vi "单参数加标流程.vi"(10 "流程类型":T3, 11 "Slave ID":T5=enum."氨氮") -> ()   [LabVIEW 2016, in "质控单元V2.lvlib"]
panel:
  in  "平行样测试数据":T1={"时间"=timestamp(0 s since 1904-01-01), "参数"="", "数据类型"="N", "第一次水样浓度值"=0.0, "第二次水样测试时间"=timestamp(0 s since 1904-01-01), "第二次水样浓度值"=0.0}
  in  "集成干预测试数据":T2={"时间"=timestamp(0 s since 1904-01-01), "参数"="", "数据类型"="N", "集成干预测试浓度值"=0.0, "集成干预前测试时间"=timestamp(0 s since 1904-01-01), "集成干预前测试浓度值"=0.0}
  out "平行样启动时间":timestamp
  in  "获取加标回收测试数据计数":u16
  in  "获取水样测试数据计数":u16
  in  "写入加标体积重试次数":u16
  in  "加标模块加标润洗启动计数":u16
  out "加标回收启动时间":timestamp
  out "水样测试启动时间":timestamp
  out "Next State":string
  in  "仪器加标回收启动计数":u16
  in  "仪器水样测试启动计数":u16
  in  "加标模块排液启动计数":u16
  in  "加标模块加标启动计数":u16
  in  "加标模块进样启动计数":u16
  in  "加标模块水样润洗启动计数":u16
  in  "采配水启动次数计数":u16
  in  "加标回收测试时间":timestamp
  in  "水样测试时间":timestamp
  in  "质控数据":T4
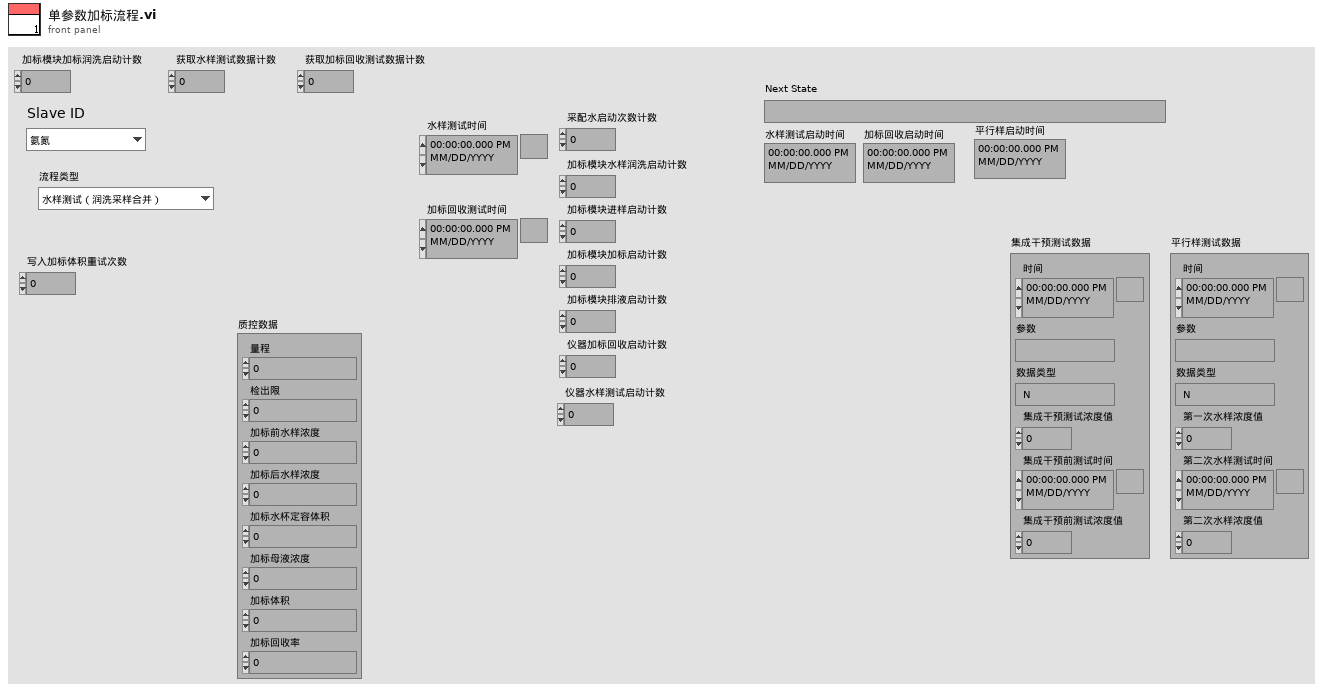
[diagram p1: front panel]
types:
  T1 = typedef "平行样测试数据字段定义.ctl" = cluster{"时间":timestamp, "参数":string, "数据类型":string, "第一次水样浓度值":dbl, "第二次水样测试时间":timestamp, "第二次水样浓度值":dbl}
  T2 = typedef "集成干预字段定义.ctl" = cluster{"时间":timestamp, "参数":string, "数据类型":string, "集成干预测试浓度值":dbl, "集成干预前测试时间":timestamp, "集成干预前测试浓度值":dbl}
  T3 = typedef "质控单元V2.lvlib/测试子流程.ctl" = enum16{"水样测试（润洗采样合并）", "水样测试（不启动采配水）", "加标回收（润洗采样合并）", "加标回收（不启动采配水）", "集成干预测试", "平行样测试", "平行样测试（不启动采配水）", "水样测试（不含采样杯）", "平行样测试（不含采样杯）", "集成干预测试（不含采样杯）"}
  T4 = cluster{"量程":dbl, "检出限":dbl, "加标前水样浓度":dbl, "加标后水样浓度":dbl, "加标水杯定容体积":dbl, "加标母液浓度":dbl, "加标体积":dbl, "加标回收率":dbl}
  T5 = typedef "质控单元V2.lvlib/质控slave id.ctl" = enum16{"null", "氨氮", "总磷", "总氮", "CODMn", "CODCr"}
  T6 = cluster{"氨氮":bool, "总磷":bool, "总氮":bool, "CODMn":bool, "CODCr":bool}
  T7 = cluster{"时间":timestamp, "参数":string, "数据类型":string, "加标回收率":sgl, "加标前水样测试时间":timestamp, "加标前水样浓度值":sgl, "加标后水样浓度值":sgl, "加标母液浓度值":sgl, "加标体积":sgl, "加标水杯定容体积":sgl}
  T8 = enum16{"待机", "水样测试（全流程）", "停止", "加标回收", "水样测试（简易流程）"}
  T9 = enum16{"待机", "润洗", "采样", "沉淀", "配水", "反冲洗", "储水", "结束"}
  T10 = typedef "质控单元V2.lvlib/采配水通用流程.ctl" = enum16{"待机", "润洗", "采样", "沉淀", "配水", "反冲洗", "结束"}
  T11 = typedef "质控单元V2.lvlib/质控流程控制.ctl" = enum16{"待机", "启动进样流程", "启动加标流程", "启动排液流程", "停止流程", "加标（单独一步骤）"}
  T12 = enum16{"待机", "润洗", "进样", "定量", "加标", "等待取样", "排液", "异常停机"}
  T13 = enum16{"空闲", "水样测试", "标样核查", "零点核查", "跨度核查", "空白测试", "平行样测试", "加标回收", "空白校准", "标样校准", "初始化（清洗）"}
  T14 = cluster{"时间":timestamp, "参数":string, "数据类型":string, "第一次水样浓度值":dbl, "第二次水样测试时间":timestamp, "第二次水样浓度值":dbl}
  T15 = cluster{"水样数据时间":timestamp, "水样实测值":sgl, "水样数据标识":string}
  T16 = cluster{"加标回收数据时间":timestamp, "加标回收实测值":sgl, "加标回收数据标识":string}
  T17 = typedef "质控单元V2.lvlib/质控仪器状态.ctl" = cluster{"运行状态":enum16{"待机", "润洗", "进样", "定量", "加标", "等待取样", "排液"}, "液位状态":enum16{"无感应", "有感应"}, "告警状态":enum16{"无告警", "液位故障告警", "注射泵异常"}, "当前步骤数":u16, "当前步骤剩余时间":u16, "当前步骤具体操作":enum16{"加标", "进样", "排液", "搅拌", "定量"}, "当前流程":enum16{"待机", "进样流程", "加标流程", "排液流程"}}
  T18 = enum16{"待机", "润洗", "进样", "定量", "加标", "等待取样", "排液"}
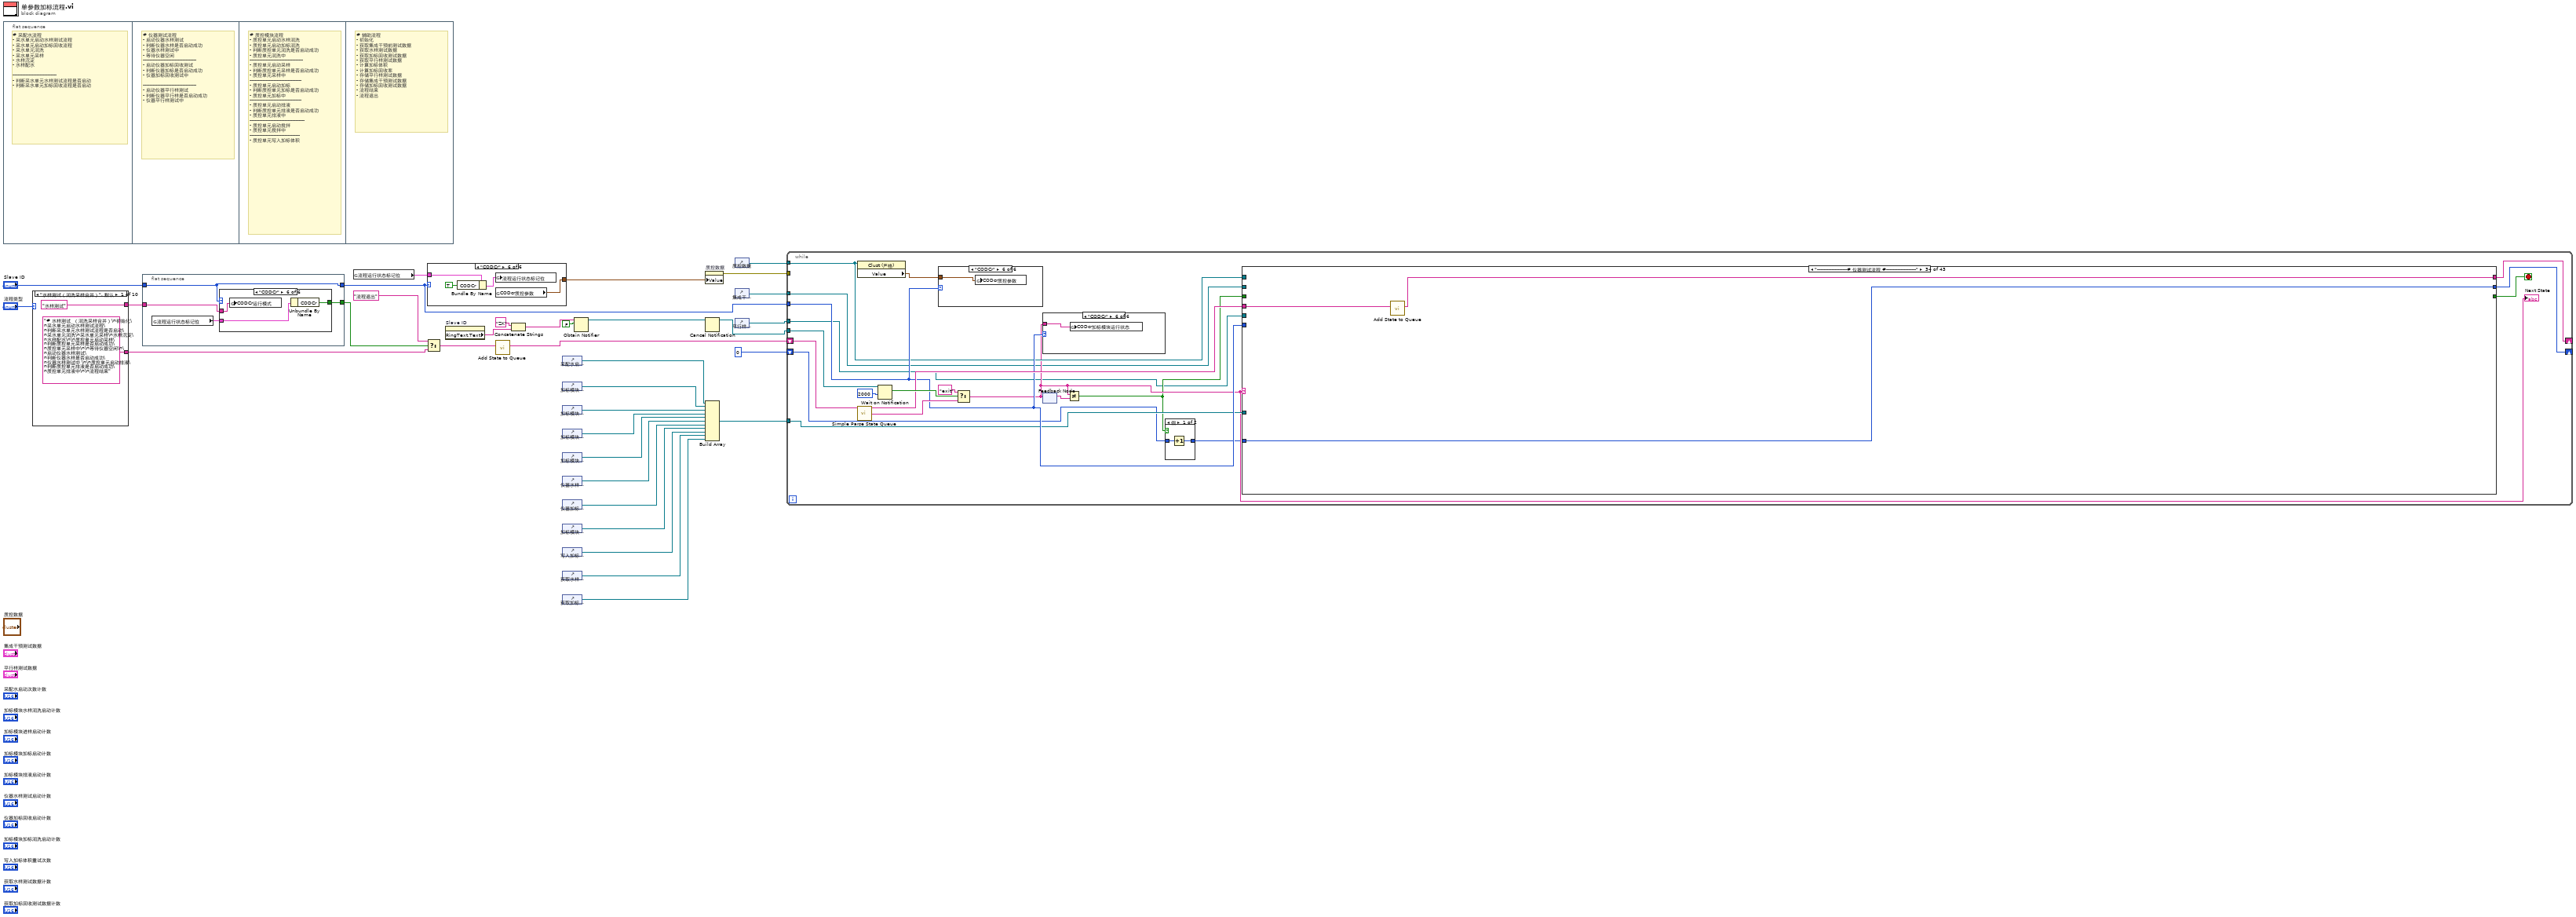
[diagram p0: block diagram]
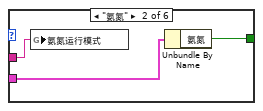
[diagram p3: hidden frame]
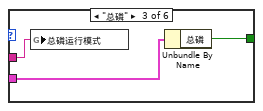
[diagram p4: hidden frame]
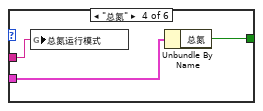
[diagram p5: hidden frame]
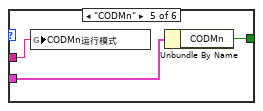
[diagram p6: hidden frame]
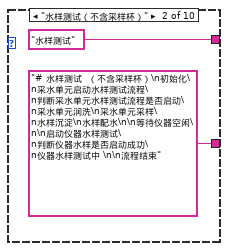
[diagram p7: hidden frame]
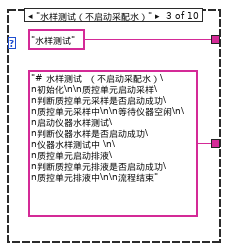
[diagram p8: hidden frame]
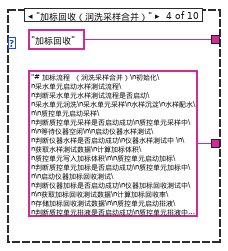
[diagram p9: hidden frame]
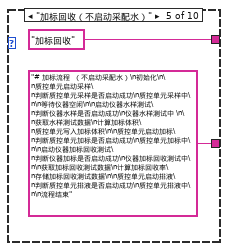
[diagram p10: hidden frame]
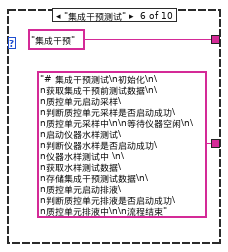
[diagram p11: hidden frame]
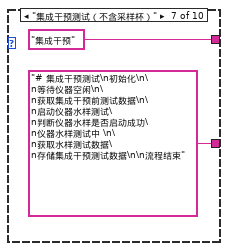
[diagram p12: hidden frame]
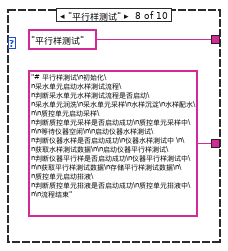
[diagram p13: hidden frame]
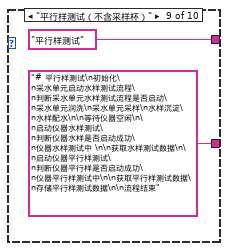
[diagram p14: hidden frame]
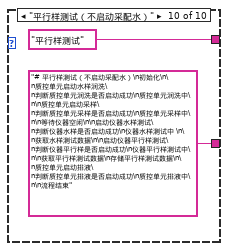
[diagram p15: hidden frame]
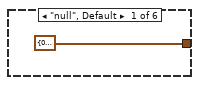
[diagram p16: hidden frame]
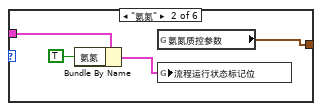
[diagram p17: hidden frame]
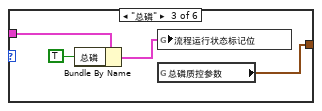
[diagram p18: hidden frame]
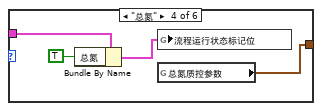
[diagram p19: hidden frame]
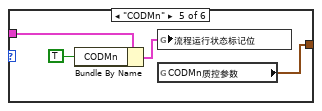
[diagram p20: hidden frame]
diagram:
  n1 = flat-sequence {
    frame #0 {
      # "# 采配水流程\n- 采水单元启动水样测试流程\n- 采水单元启动加标回收流程\n- 采水单元润洗\n- 采水单元采样 \n- 水样沉淀\n- 水样配水\n\n----------------------------\n- 判断采水单元水样测试流程是否启动\n- 判断采水单元加标回收流程是否启动"
    }
    frame #1 {
      # "# 仪器测试流程\n- 启动仪器水样测试\n- 判断仪器水样是否启动成功\n- 仪器水样测试中\n- 等待仪器空闲\n----------------------------------\n- 启动仪器加标回收测试\n- 判断仪器加标是否启动成功\n- 仪器加标回收测试中\n\n----------------------------------\n- 启动仪器平行样测试\n- 判断仪器平行样是否启动成功\n- 仪器平行样测试中"
    }
    frame #2 {
      # "# 质控模块流程\n- 质控单元启动水样润洗\n- 质控单元启动加标润洗\n- 判断质控单元润洗是否启动成功\n- 质控单元润洗中\n----------------------------------\n- 质控单元启动采样\n- 判断质控单元采样是否启动成功\n- 质控单元采样中\n---------------------------------\n- 质控单元启动加标\n- 判断质控单元加标是否启动成功\n- 质控单元加标中\n---------------------------------\n- 质控单元启动排液\n- 判断质控单元排液是否启动成功\n- 质控单元排液中\n-----------------------------------\n- 质控单元启动搅拌\n- 质控单元搅拌中\n--------------------------------\n- 质控单元写入加标体积"
    }
    frame #3 {
      # "# 辅助流程\n- 初始化\n- 获取集成干预前测试数据\n- 获取水样测试数据\n- 获取加标回收测试数据\n- 获取平行样测试数据\n- 计算加标体积\n- 计算加标回收率\n- 存储平行样测试数据\n- 存储集成干预测试数据\n- 存储加标回收测试数据 \n- 流程结束\n- 流程退出"
    }
  }
  n2 = case shown="\"水样测试（润洗采样合并）\", 默认" "流程类型" {
    tunnel: ["# 水样测试  （润洗采样合并）\n初始化\n采水单元启动水样测试流程\n判断采水单元水样测试流程是否启动\n采水单元润洗\n采水单元采样\n水样沉淀\n水样配水\n\n质控单元启动采样\n判断质控单元采样是否启动成功\n质控单元采样中\n\n等待仪器空闲\n\n启动仪器水样测试\n判断仪器水样是否启动成功\n仪器水样测试中 \n\n质控单元启动排液\n判断质控单元排液是否启动成功\n质控单元排液中\n\n流程结束" ("State(s) In (\"\")") "# 水样测试  （不含采样杯）\n初始化\n采水单元启动水样测试流程\n判断采水单元水样测试流程是否启动\n采水单元润洗\n采水单元采样\n水样沉淀\n水样配水\n\n等待仪器空闲\n\n启动仪器水样测试\n判断仪器水样是否启动成功\n仪器水样测试中 \n\n流程结束" ("State(s) In (\"\")") "# 水样测试  （不启动采配水）\n初始化\n\n质控单元启动采样\n判断质控单元采样是否启动成功\n质控单元采样中\n\n等待仪器空闲\n\n启动仪器水样测试\n判断仪器水样是否启动成功\n仪器水样测试中 \n\n质控单元启动排液\n判断质控单元排液是否启动成功\n质控单元排液中\n\n流程结束" ("State(s) In (\"\")") "# 加标流程  （润洗采样合并）\n初始化\n采水单元启动水样测试流程\n判断采水单元水样测试流程是否启动\n采水单元润洗\n采水单元采样\n水样沉淀\n水样配水\n\n质控单元启动采样\n判断质控单元采样是否启动成功\n质控单元采样中\n\n等待仪器空闲\n\n启动仪器水样测试\n判断仪器水样是否启动成功\n仪器水样测试中 \n\n获取水样测试数据\n计算加标体积\n质控单元写入加标体积\n\n质控单元启动加标\n判断质控单元加标是否启动成功\n质控单元加标中\n\n启动仪器加标回收测试\n判断仪器加标是否启动成功\n仪器加标回收测试中\n\n获取加标回收测试数据\n计算加标回收率\n存储加标回收测试数据\n\n质控单元启动排液\n判断质控单元排液是否启动成功\n质控单元排液中\n\n流程结束" ("State(s) In (\"\")") "# 加标流程  （不启动采配水）\n初始化\n\n质控单元启动采样\n判断质控单元采样是否启动成功\n质控单元采样中\n\n等待仪器空闲\n\n启动仪器水样测试\n判断仪器水样是否启动成功\n仪器水样测试中 \n\n获取水样测试数据\n计算加标体积\n质控单元写入加标体积\n\n质控单元启动加标\n判断质控单元加标是否启动成功\n质控单元加标中\n\n启动仪器加标回收测试\n判断仪器加标是否启动成功\n仪器加标回收测试中\n\n获取加标回收测试数据\n计算加标回收率\n存储加标回收测试数据\n\n质控单元启动排液\n判断质控单元排液是否启动成功\n质控单元排液中\n\n流程结束" ("State(s) In (\"\")") "# 集成干预测试\n初始化\n\n获取集成干预前测试数据\n\n质控单元启动采样\n判断质控单元采样是否启动成功\n质控单元采样中\n\n等待仪器空闲\n\n启动仪器水样测试\n判断仪器水样是否启动成功\n仪器水样测试中 \n\n获取水样测试数据\n存储集成干预测试数据\n\n质控单元启动排液\n判断质控单元排液是否启动成功\n质控单元排液中\n\n流程结束" ("State(s) In (\"\")") "# 集成干预测试\n初始化\n\n等待仪器空闲\n\n获取集成干预前测试数据\n\n启动仪器水样测试\n判断仪器水样是否启动成功\n仪器水样测试中 \n\n获取水样测试数据\n存储集成干预测试数据\n\n流程结束" ("State(s) In (\"\")") "# 平行样测试\n初始化\n采水单元启动水样测试流程\n判断采水单元水样测试流程是否启动\n采水单元润洗\n采水单元采样\n水样沉淀\n水样配水\n\n质控单元启动采样\n判断质控单元采样是否启动成功\n质控单元采样中\n\n等待仪器空闲\n\n启动仪器水样测试\n判断仪器水样是否启动成功\n仪器水样测试中 \n\n获取水样测试数据\n\n启动仪器平行样测试\n判断仪器平行样是否启动成功\n仪器平行样测试中\n\n获取平行样测试数据\n存储平行样测试数据\n\n质控单元启动排液\n判断质控单元排液是否启动成功\n质控单元排液中\n\n流程结束" ("State(s) In (\"\")") "# 平行样测试\n初始化\n采水单元启动水样测试流程\n判断采水单元水样测试流程是否启动\n采水单元润洗\n采水单元采样\n水样沉淀\n水样配水\n\n等待仪器空闲\n\n启动仪器水样测试\n判断仪器水样是否启动成功\n仪器水样测试中 \n\n获取水样测试数据\n\n启动仪器平行样测试\n判断仪器平行样是否启动成功\n仪器平行样测试中\n\n获取平行样测试数据\n存储平行样测试数据\n\n流程结束" ("State(s) In (\"\")") "# 平行样测试（不启动采配水）\n初始化\n\n质控单元启动水样润洗\n判断质控单元润洗是否启动成功\n质控单元润洗中\n\n质控单元启动采样\n判断质控单元采样是否启动成功\n质控单元采样中\n\n等待仪器空闲\n\n启动仪器水样测试\n判断仪器水样是否启动成功\n仪器水样测试中 \n\n获取水样测试数据\n\n启动仪器平行样测试\n判断仪器平行样是否启动成功\n仪器平行样测试中\n\n获取平行样测试数据\n存储平行样测试数据\n\n质控单元启动排液\n判断质控单元排液是否启动成功\n质控单元排液中\n\n流程结束" ("State(s) In (\"\")")] -> w12
    tunnel: ["水样测试" "水样测试" "水样测试" "加标回收" "加标回收" "集成干预" "集成干预" "平行样测试" "平行样测试" "平行样测试"] -> w6
    frame "水样测试（润洗采样合并）", Default {
    }
    frame "水样测试（不含采样杯）" {
    }
    frame "水样测试（不启动采配水）" {
    }
    frame "加标回收（润洗采样合并）" {
    }
    frame "加标回收（不启动采配水）" {
    }
    frame "集成干预测试" {
    }
    frame "集成干预测试（不含采样杯）" {
    }
    frame "平行样测试" {
    }
    frame "平行样测试（不含采样杯）" {
    }
    frame "平行样测试（不启动采配水）" {
    }
  }
  n3 = flat-sequence {
    tunnel: [w56] -> w15
    tunnel: [w57] -> w14
    tunnel: "Slave ID" -> [w56]
    tunnel: w6 -> [w55]
    frame #0 {
      n4 = global read "ZK非断电保存全局变量.vi" "流程运行状态标记位"() -> (w58:T6)
      n5 = case shown="\"CODCr\"" w56 {
        tunnel: w58 -> [_ w61 w64 w67 w70 w73]
        tunnel: [_ w60 w63 w66 w69 w72] -> w57
        tunnel: w55 -> [_ w59 w62 w65 w68 w71]
        frame "null", Default {
        }
        frame "氨氮" {
          n6 = global write "ZK非断电保存全局变量.vi" "氨氮运行模式"(w59) -> ()
          n7 = Unbundle By Name(w61) -> ("氨氮"=w60:bool)
        }
        frame "总磷" {
          n8 = global write "ZK非断电保存全局变量.vi" "总磷运行模式"(w62) -> ()
          n9 = Unbundle By Name(w64) -> ("总磷"=w63:bool)
        }
        frame "总氮" {
          n10 = global write "ZK非断电保存全局变量.vi" "总氮运行模式"(w65) -> ()
          n11 = Unbundle By Name(w67) -> ("总氮"=w66:bool)
        }
        frame "CODMn" {
          n12 = global write "ZK非断电保存全局变量.vi" "CODMn运行模式"(w68) -> ()
          n13 = Unbundle By Name(w70) -> ("CODMn"=w69:bool)
        }
        frame "CODCr" {
          n14 = global write "ZK非断电保存全局变量.vi" "CODCr运行模式"(w71) -> ()
          n15 = Unbundle By Name(w73) -> ("CODCr"=w72:bool)
        }
      }
    }
  }
  n16 = global read "ZK非断电保存全局变量.vi" "流程运行状态标记位"() -> (w17:T6)
  n17 = Select(t="流程退出", s=w14, f=w12) -> (s? t:f=w11:string)
  n18 = case shown="\"CODCr\"" w15 {
    tunnel: [T4 {"量程"=0.0, "检出限"=0.0, "加标前水样浓度"=0.0, "加标后水样浓度"=0.0, "加标水杯定容体积"=0.0, "加标母液浓度"=0.0, "加标体积"=0.0, "加标回收率"=0.0} ("CODcr质控参数") w78 w82 w86 w90 w94] -> w26
    tunnel: w17 -> [_ w77 w79 w83 w87 w91]
    frame "null", Default {
    }
    frame "氨氮" {
      n19 = Bundle By Name(cluster=w77, "氨氮"=TRUE) -> (w76:T6)
      n20 = global read "ZK断电保存全局变量.vi" "氨氮质控参数"() -> (w78:T4)
      n21 = global write "ZK非断电保存全局变量.vi" "流程运行状态标记位"(w76) -> ()
    }
    frame "总磷" {
      n22 = Bundle By Name(cluster=w79, "总磷"=TRUE ("氨氮")) -> (w81:T6)
      n23 = global write "ZK非断电保存全局变量.vi" "流程运行状态标记位"(w81) -> ()
      n24 = global read "ZK断电保存全局变量.vi" "总磷质控参数"() -> (w82:T4)
    }
    frame "总氮" {
      n25 = Bundle By Name(cluster=w83, "总氮"=TRUE ("氨氮")) -> (w85:T6)
      n26 = global write "ZK非断电保存全局变量.vi" "流程运行状态标记位"(w85) -> ()
      n27 = global read "ZK断电保存全局变量.vi" "总氮质控参数"() -> (w86:T4)
    }
    frame "CODMn" {
      n28 = Bundle By Name(cluster=w87, "CODMn"=TRUE ("氨氮")) -> (w89:T6)
      n29 = global write "ZK非断电保存全局变量.vi" "流程运行状态标记位"(w89) -> ()
      n30 = global read "ZK断电保存全局变量.vi" "CODMn质控参数"() -> (w90:T4)
    }
    frame "CODCr" {
      n31 = Bundle By Name(cluster=w91, "CODCr"=TRUE ("氨氮")) -> (w93:T6)
      n32 = global write "ZK非断电保存全局变量.vi" "流程运行状态标记位"(w93) -> ()
      n33 = global read "ZK断电保存全局变量.vi" "CODcr质控参数"() -> (w94:T4)
    }
  }
  n34 = property on="Slave ID" class="Enum (严格)"() -> ("RingText.Text"=w34:string)  [unwired: 2 in, 2 out]
  n35 = call "Add State to Queue.vi"("State(s) In (\"\")"=w11) -> ("States Out"=w28:string)  [unwired: 14 in]
  n36 = Concatenate Strings("ZK" ("字符串"), w34) -> (w32:string)
  n37 = control-ref of="采配水启动次数计数"() -> (w24:refnum<vi>)
  n38 = control-ref of="加标模块水样润洗启动计数"() -> (w23:refnum<vi>)
  n39 = control-ref of="加标模块进样启动计数"() -> (w22:refnum<vi>)
  n40 = control-ref of="加标模块加标启动计数"() -> (w21:refnum<vi>)
  n41 = control-ref of="加标模块排液启动计数"() -> (w20:refnum<vi>)
  n42 = control-ref of="仪器水样测试启动计数"() -> (w4:refnum<vi>)
  n43 = control-ref of="仪器加标回收启动计数"() -> (w5:refnum<vi>)
  n44 = control-ref of="加标模块加标润洗启动计数"() -> (w16:refnum<vi>)
  n45 = control-ref of="写入加标体积重试次数"() -> (w10:refnum<vi>)
  n46 = control-ref of="获取水样测试数据计数"() -> (w9:refnum<vi>)
  n47 = control-ref of="获取加标回收测试数据计数"() -> (w8:refnum<vi>)
  n48 = Obtain Notifier(name (unnamed)=w32, notification data type=FALSE) -> (notifier out=w30:refnum<notifier>)  [unwired: 2 in, 2 out]
  n49 = property on="质控数据" class="Clust (严格)"("Value"=w26) -> (error out=w27:errorcluster)  [unwired: 2 in, 1 out]
  n50 = Cancel Notification(0:w30) -> (8:w29:refnum<notifier>)  [unwired: 1 in, 2 out]
  n51 = Build Array(w24, w23, w22, w21, w20, w4, w5, w16, w10, w9, w8) -> (w19:refnum<vi>[])
  n52 = control-ref of="质控数据"() -> (w25:refnum<vi>)
  n53 = control-ref of="集成干预测试数据"() -> (w2:refnum<vi>)
  n54 = control-ref of="平行样测试数据"() -> (w1:refnum<vi>)
  n55 = while {
    tunnel: w29 -> [w114]
    tunnel: w15 -> [w106]
    shift-right: [w108] -> _
    shift-left: w28 -> [w115]
    tunnel: w27 -> [_]
    tunnel: w25 -> [w105]
    tunnel: w19 -> [w103]
    shift-right: [w98] -> _
    shift-left: 0 -> [w100]
    tunnel: w2 -> [w95]
    tunnel: w1 -> [w96]
    stop <- w107 stop-if-true
    n56 = property class="Clust (严格)"(reference=w105) -> ("Value"=w104:T4)  [unwired: 1 in, 2 out]
    n57 = call "Simple Parse State Queue.vi"("State Queue"=w115) -> ("Remain States"=w109:string, "Next State"=w111:string)  [unwired: 13 in]
    n58 = Wait on Notification(notifier=w114, timeout in ms (-1)=2000 ("超时毫秒(-1)")) -> (notification=w112:bool)  [unwired: 2 in, 3 out]
    n59 = case shown="\"CODCr\"" w106 {
      tunnel: w104 -> [_ w118 w119 w120 w121 w122]
      frame "null", Default {
      }
      frame "氨氮" {
        n60 = global write "ZK断电保存全局变量.vi" "氨氮质控参数"(w118) -> ()
      }
      frame "总磷" {
        n61 = global write "ZK断电保存全局变量.vi" "总磷质控参数"(w119) -> ()
      }
      frame "总氮" {
        n62 = global write "ZK断电保存全局变量.vi" "总氮质控参数"(w120) -> ()
      }
      frame "CODMn" {
        n63 = global write "ZK断电保存全局变量.vi" "CODMn质控参数"(w121) -> ()
      }
      frame "CODCr" {
        n64 = global write "ZK断电保存全局变量.vi" "CODcr质控参数"(w122) -> ()
      }
    }
    n65 = Select(t="exit" ("State(s) In (\"\")"), s=w112, f=w111) -> (s? t:f=w101:string)
    "Next State" <- w101
    n66 = case shown="\"CODCr\"" w106 {
      tunnel: w101 -> [_ w123 w124 w125 w126 w127]
      frame "null", Default {
      }
      frame "氨氮" {
        n67 = global write "ZK非断电保存全局变量.vi" "氨氮加标模块运行状态"(w123) -> ()
      }
      frame "总磷" {
        n68 = global write "ZK非断电保存全局变量.vi" "总磷加标模块运行状态"(w124) -> ()
      }
      frame "总氮" {
        n69 = global write "ZK非断电保存全局变量.vi" "总氮加标模块运行状态"(w125) -> ()
      }
      frame "CODMn" {
        n70 = global write "ZK非断电保存全局变量.vi" "CODMn加标模块运行状态"(w126) -> ()
      }
      frame "CODCr" {
        n71 = global write "ZK非断电保存全局变量.vi" "CODcr加标模块运行状态"(w127) -> ()
      }
    }
    n72 = feedback-in #1(w101) -> ()
    n73 = feedback #1() -> (w102:string)  [unwired: 1 in]
    n74 = Not Equal?(x=w101, y=w102) -> (x != y?=w97:bool)
    n75 = case shown="假" w97 {
      tunnel: w100 -> [w117 _]
      tunnel: [w116 _] -> w99
      frame False {
        n76 = Increment(x=w117) -> (x+1=w116:i32)
      }
      frame True {
      }
    }
    n77 = case shown="\"-------------------# 仪器测试流程 #-------------------\"" w101 {
      selector: w101 -> [_ _ w139 w164 w221 w231 w285 w336 w346 w357 w384 w401 w413 w443 _ w453 w464 w476 w497 w519 w540 w561 w583 _ w600 w618 w638 w650 w662 w701 w740 w789 w821 _ w853 w870 w893 w911 w930 w966 w1004 w1044 w1084]
      tunnel: w109 -> [w130 w133 w148 w186 w223 w257 w309 w344 w353 w371 w387 w403 w419 w447 w450 w461 w472 w491 w498 w531 w549 w569 w591 w598 w610 w625 w648 w660 w684 w723 w762 w798 w831 w849 w862 w874 w902 w920 w932 w983 w1022 w1061 w1090]
      tunnel: [w129 w132 w147 w185 w222 w256 w308 w343 w352 w370 w386 w402 w418 w446 w449 w460 w471 w490 w512 w530 w548 w568 w590 w597 w609 w624 w647 w659 w683 w722 w761 w797 w830 w848 w861 w873 w901 w919 w931 w982 w1021 w1060 w1089] -> w108
      tunnel: [_ _ _ _ _ _ _ _ _ _ _ _ TRUE TRUE _ _ _ _ _ _ _ _ _ _ _ _ _ _ _ _ _ _ _ _ _ _ _ _ _ _ _ _ _] -> w107
      tunnel: w106 -> [_ _ w138 w173 w215 w242 w296 w335 w347 w358 w385 w396 w414 w444 _ w454 w465 w475 w496 w518 w538 w558 w581 _ w601 w612 w639 w651 w669 w708 w747 w783 w819 _ w854 w871 w894 w912 w928 w969 w1008 w1047 w1083]
      tunnel: w105 -> [_ _ w144 w184 _ w255 _ w342 w351 w369 _ _ _ _ _ _ _ _ _ _ _ _ _ _ _ w623 _ _ _ _ _ _ _ _ _ _ _ _ _ _ _ _ _]
      tunnel: w103 -> [_ _ w135 w170 _ w233 w287 _ _ _ _ _ _ _ _ w459 w470 w480 w502 _ _ _ _ _ w603 w617 w642 w654 w674 w713 w752 _ _ _ w857 _ w897 w915 _ w974 w1014 w1053 _]
      tunnel: w99 -> [w128 w131 w134 w161 w220 w230 w284 w334 w345 w354 w383 w400 w410 w440 w448 w452 w463 w473 w494 w516 w537 w556 w580 w596 w599 w611 w637 w649 w667 w707 w745 w781 w817 w847 w851 w872 w891 w909 w927 w968 w1007 w1046 w1080]
      tunnel: [w128 w131 w134 w161 w220 w230 w284 w334 w345 w354 w383 w400 w410 w440 w448 w452 w463 w473 w494 w516 w537 w556 w580 w596 w599 w611 w637 w649 w667 w707 w745 w781 w817 w847 w851 w872 w891 w909 w927 w968 w1007 w1046 w1080] -> w98
      tunnel: w97 -> [_ _ _ _ _ _ _ _ _ _ _ _ _ _ _ _ _ _ _ w515 w536 w555 w579 _ _ _ _ _ w668 w706 w746 w782 w818 _ _ w868 _ _ _ w965 w1005 w1043 w1081]
      tunnel: w96 -> [_ _ _ w159 _ _ w283 _ _ _ w382 _ _ _ _ _ _ _ _ _ _ _ _ _ _ _ _ _ _ _ _ _ _ _ _ _ _ _ _ _ _ _ _]
      tunnel: w95 -> [_ _ _ w153 w216 _ _ _ _ _ _ w399 _ _ _ _ _ _ _ _ _ _ _ _ _ _ _ _ _ _ _ _ _ _ _ _ _ _ _ _ _ _ _]
      frame Default {
        n78 = call "Add State to Queue.vi"("State(s) In (\"\")"=w130) -> ("States Out"=w129:string)  [unwired: 14 in]
      }
      frame "-------------------# 辅助流程 #-------------------" {
        n79 = call "Add State to Queue.vi"("State(s) In (\"\")"=w133) -> ("States Out"=w132:string)  [unwired: 14 in]
      }
      frame "初始化" {
        w140 = 0.0 ("加标前水样浓度")
        n80 = call "ZK报警清除.vi"("Slave ID"=w138) -> ()  [unwired: 10 in, 1 out]
        n81 = local write "加标回收测试时间"(timestamp(0 s since 1904-01-01) ("加标回收测试时间")) -> ()
        n82 = for {
          tunnel: w135 -> [w150] mode=indexing
          n83 = property class="DigNum (严格)"(reference=w150, "Value"=u16 0 ("值")) -> ()  [unwired: 1 in, 2 out]
        }
        n84 = property class="Clust (严格)"(reference=w144) -> (reference out=w143:refnum<vi>, "Value"=w142:T4)  [unwired: 1 in, 1 out]
        n85 = Concatenate Strings("----->>" ("字符串"), w139) -> (w137:string)
        n86 = local write "水样测试时间"(timestamp(0 s since 1904-01-01) ("水样测试时间")) -> ()
        n87 = call "启动日志.vi"("日志信息"=w137, "Slave ID"=w138) -> ()  [unwired: 9 in, 1 out]
        n88 = Bundle By Name(cluster=w142, "加标前水样浓度"=w140, "加标后水样浓度"=w140, "加标体积"=w140, "加标回收率"=w140) -> (w141:T4)
        n89 = property class="Clust (严格)"(reference=w143, "Value"=w141) -> ()  [unwired: 1 in, 2 out]
        n90 = call "Add State to Queue.vi"("State(s) In (\"\")"=w148) -> ("States Out"=w147:string)  [unwired: 14 in]
      }
      frame "获取水样测试数据" {
        n91 = call "启动日志.vi"("日志信息"=w164, "Slave ID"=w173) -> ()  [unwired: 9 in, 1 out]
        n92 = property class="Clust (严格)"(reference=w159) -> (reference out=w160:refnum<vi>, "Value"=w158:T14)  [unwired: 1 in, 1 out]
        n93 = case shown="\"CODCr\"" w173 {
          tunnel: [sgl 0.0 ("水样实测值") w194 w198 w202 w206 w210] -> w151
          tunnel: [timestamp(0 s since 1904-01-01) ("水样数据时间") w193 w197 w201 w205 w209] -> w152
          frame "null", Default {
          }
          frame "氨氮" {
            w191 = u16 3 items=["总磷"=1, "总氮"=2, "氨氮"=3, "CODMn"=21, "CODcr"=22] ("站号")
            n94 = call-poly "获取测试数据.vi"("站号"=w191) -> ("测量数据区"=w192:T15)  [unwired: 10 in]
            n95 = Unbundle By Name(w192) -> ("水样数据时间"=w193:timestamp, "水样实测值"=w194:sgl)
          }
          frame "总磷" {
            w195 = u16 1 items=["总磷"=1, "总氮"=2, "氨氮"=3, "CODMn"=21, "CODcr"=22] ("站号")
            n96 = call-poly "获取测试数据.vi"("站号"=w195) -> ("测量数据区"=w196:T15)  [unwired: 10 in]
            n97 = Unbundle By Name(w196) -> ("水样数据时间"=w197:timestamp, "水样实测值"=w198:sgl)
          }
          frame "总氮" {
            w199 = u16 2 items=["总磷"=1, "总氮"=2, "氨氮"=3, "CODMn"=21, "CODcr"=22] ("站号")
            n98 = call-poly "获取测试数据.vi"("站号"=w199) -> ("测量数据区"=w200:T15)  [unwired: 10 in]
            n99 = Unbundle By Name(w200) -> ("水样数据时间"=w201:timestamp, "水样实测值"=w202:sgl)
          }
          frame "CODMn" {
            w203 = u16 21 items=["总磷"=1, "总氮"=2, "氨氮"=3, "CODMn"=21, "CODcr"=22] ("站号")
            n100 = call-poly "获取测试数据.vi"("站号"=w203) -> ("测量数据区"=w204:T15)  [unwired: 10 in]
            n101 = Unbundle By Name(w204) -> ("水样数据时间"=w205:timestamp, "水样实测值"=w206:sgl)
          }
          frame "CODCr" {
            w207 = u16 22 items=["总磷"=1, "总氮"=2, "氨氮"=3, "CODMn"=21, "CODcr"=22] ("站号")
            n102 = call-poly "获取测试数据.vi"("站号"=w207) -> ("测量数据区"=w208:T15)  [unwired: 10 in]
            n103 = Unbundle By Name(w208) -> ("水样数据时间"=w209:timestamp, "水样实测值"=w210:sgl)
          }
        }
        n104 = property class="Clust (严格)"(reference=w153) -> (reference out=w154:refnum<vi>, "Value"=w155:T2)  [unwired: 1 in, 1 out]
        n105 = property class="Clust (严格)"(reference=w184) -> (reference out=w183:refnum<vi>, "Value"=w182:T4)  [unwired: 1 in, 1 out]
        n106 = Index Array(array=w170, index=9 ("索引")) -> (element=w171:refnum<vi>)
        n107 = property class="DigNum (严格)"(reference=w171) -> (reference out=w169:refnum<vi>, "Value"=w168:u16)  [unwired: 1 in, 1 out]
        n108 = Increment(x=w168) -> (x+1=w167:u16)
        n109 = property class="DigNum (严格)"(reference=w169, "Value"=w167) -> ()  [unwired: 1 in, 2 out]
        n110 = Less Or Equal?(x=w167, y=u16 5) -> (x <= y?=w165:bool)
        n111 = Select(t=w164, s=w165, f="exit") -> (s? t:f=w162:string)
        n112 = local write "水样测试时间"(w152) -> ()
        n113 = local read "水样测试启动时间"() -> (w180:timestamp)
        n114 = Subtract(x=w152, y=w180) -> (x-y=w179:dbl)
        n115 = Bundle By Name(cluster=w158, "时间"=w152, "第一次水样浓度值"=w151) -> (w157:T14)
        n116 = Bundle By Name(cluster=w155, "时间"=w152, "集成干预测试浓度值"=w151) -> (w156:T2)
        n117 = Bundle By Name(cluster=w182, "加标前水样浓度"=w151) -> (w181:T4)
        n118 = Absolute Value(x=w179) -> (abs(x)=w178:dbl)
        n119 = property class="Clust (严格)"(reference=w160, "Value"=w157) -> ()  [unwired: 1 in, 2 out]
        n120 = property class="Clust (严格)"(reference=w154, "Value"=w156) -> ()  [unwired: 1 in, 2 out]
        n121 = property class="Clust (严格)"(reference=w183, "Value"=w181) -> ()  [unwired: 1 in, 2 out]
        n122 = Less?(x=w178, y=300.0) -> (x < y?=w174:bool)
        n123 = case shown="假" w174 {
          tunnel: w173 -> [w188 _]
          frame False {
            w187 = "获取水样数据异常" ("日志信息")
            n124 = call "启动日志.vi"("日志信息"=w187, "Slave ID"=w188) -> ()  [unwired: 9 in, 1 out]
            n125 = call "报警信息记录.vi"("报警信息"=w187, "Slave ID"=w188) -> ()  [unwired: 9 in, 1 out]
          }
          frame True {
          }
        }
        n126 = Select(t="", s=w174, f=w162) -> (s? t:f=w175:string)
        n127 = call "Add State to Queue.vi"("State(s) In Front (\"\")"=w175, "State(s) In (\"\")"=w186) -> ("States Out"=w185:string)  [unwired: 13 in]
      }
      frame "获取集成干预前测试数据" {
        n128 = call "启动日志.vi"("日志信息"=w221, "Slave ID"=w215) -> ()  [unwired: 9 in, 1 out]
        n129 = property class="Clust (严格)"(reference=w216) -> (reference out=w217:refnum<vi>, "Value"=w218:T2)  [unwired: 1 in, 1 out]
        n130 = case shown="\"CODMn\"" w215 {
          tunnel: ["" "氨氮" "总磷" "总氮" "CODMn" "CODCr"] -> w214
          frame "null", Default {
          }
          frame "氨氮" {
          }
          frame "总磷" {
          }
          frame "总氮" {
          }
          frame "CODMn" {
          }
          frame "CODCr" {
          }
        }
        n131 = call "Add State to Queue.vi"("State(s) In (\"\")"=w223) -> ("States Out"=w222:string)  [unwired: 14 in]
        n132 = call "获取最新一笔数据.vi"("table"=w214) -> ("检测值"=w213:cluster{"时间":timestamp, "检测值":dbl})  [unwired: 8 in, 2 out]
        n133 = Unbundle By Name(w213) -> ("时间"=w212:timestamp, "检测值"=w211:dbl)
        n134 = Bundle By Name(cluster=w218, "集成干预前测试时间"=w212, "集成干预前测试浓度值"=w211) -> (w219:T2)
        n135 = property class="Clust (严格)"(reference=w217, "Value"=w219) -> ()  [unwired: 1 in, 2 out]
      }
      frame "获取加标回收测试数据" {
        n136 = call "启动日志.vi"("日志信息"=w231, "Slave ID"=w242) -> ()  [unwired: 9 in, 1 out]
        n137 = case shown="\"CODCr\"" w242 {
          tunnel: [sgl 0.0 ("水样实测值") w265 w269 w273 w277 w281] -> w251
          tunnel: [timestamp(0 s since 1904-01-01) ("加标回收数据时间") w264 w268 w272 w276 w280] -> w248
          frame "null", Default {
          }
          frame "氨氮" {
            w262 = u16 3 items=["总磷"=1, "总氮"=2, "氨氮"=3, "CODMn"=21, "CODcr"=22] ("站号")
            n138 = call-poly "获取测试数据.vi"("站号"=w262) -> ("测量数据区"=w263:T16)  [unwired: 10 in]
            n139 = Unbundle By Name(w263) -> ("加标回收数据时间"=w264:timestamp, "加标回收实测值"=w265:sgl)
          }
          frame "总磷" {
            w266 = u16 1 items=["总磷"=1, "总氮"=2, "氨氮"=3, "CODMn"=21, "CODcr"=22] ("站号")
            n140 = call-poly "获取测试数据.vi"("站号"=w266) -> ("测量数据区"=w267:T16)  [unwired: 10 in]
            n141 = Unbundle By Name(w267) -> ("加标回收数据时间"=w268:timestamp, "加标回收实测值"=w269:sgl)
          }
          frame "总氮" {
            w270 = u16 2 items=["总磷"=1, "总氮"=2, "氨氮"=3, "CODMn"=21, "CODcr"=22] ("站号")
            n142 = call-poly "获取测试数据.vi"("站号"=w270) -> ("测量数据区"=w271:T16)  [unwired: 10 in]
            n143 = Unbundle By Name(w271) -> ("加标回收数据时间"=w272:timestamp, "加标回收实测值"=w273:sgl)
          }
          frame "CODMn" {
            w274 = u16 21 items=["总磷"=1, "总氮"=2, "氨氮"=3, "CODMn"=21, "CODcr"=22] ("站号")
            n144 = call-poly "获取测试数据.vi"("站号"=w274) -> ("测量数据区"=w275:T16)  [unwired: 10 in]
            n145 = Unbundle By Name(w275) -> ("加标回收数据时间"=w276:timestamp, "加标回收实测值"=w277:sgl)
          }
          frame "CODCr" {
            w278 = u16 22 items=["总磷"=1, "总氮"=2, "氨氮"=3, "CODMn"=21, "CODcr"=22] ("站号")
            n146 = call-poly "获取测试数据.vi"("站号"=w278) -> ("测量数据区"=w279:T16)  [unwired: 10 in]
            n147 = Unbundle By Name(w279) -> ("加标回收数据时间"=w280:timestamp, "加标回收实测值"=w281:sgl)
          }
        }
        n148 = property class="Clust (严格)"(reference=w255) -> (reference out=w254:refnum<vi>, "Value"=w253:T4)  [unwired: 1 in, 1 out]
        n149 = Index Array(array=w233, index=10 ("索引")) -> (element=w241:refnum<vi>)
        n150 = property class="DigNum (严格)"(reference=w241) -> (reference out=w239:refnum<vi>, "Value"=w238:u16)  [unwired: 1 in, 1 out]
        n151 = Increment(x=w238) -> (x+1=w237:u16)
        n152 = property class="DigNum (严格)"(reference=w239, "Value"=w237) -> ()  [unwired: 1 in, 2 out]
        n153 = Less Or Equal?(x=w237, y=u16 5) -> (x <= y?=w235:bool)
        n154 = Select(t=w231, s=w235, f="exit") -> (s? t:f=w232:string)
        n155 = local write "加标回收测试时间"(w248) -> ()
        n156 = local read "加标回收启动时间"() -> (w249:timestamp)
        n157 = Subtract(x=w248, y=w249) -> (x-y=w247:dbl)
        n158 = Bundle By Name(cluster=w253, "加标后水样浓度"=w251) -> (w252:T4)
        n159 = Absolute Value(x=w247) -> (abs(x)=w244:dbl)
        n160 = property class="Clust (严格)"(reference=w254, "Value"=w252) -> ()  [unwired: 1 in, 2 out]
        n161 = Less?(x=w244, y=300.0) -> (x < y?=w243:bool)
        n162 = case shown="假" w243 {
          tunnel: w242 -> [w259 _]
          frame False {
            w258 = "获取加标数据异常" ("日志信息")
            n163 = call "启动日志.vi"("日志信息"=w258, "Slave ID"=w259) -> ()  [unwired: 9 in, 1 out]
            n164 = call "报警信息记录.vi"("报警信息"=w258, "Slave ID"=w259) -> ()  [unwired: 9 in, 1 out]
          }
          frame True {
          }
        }
        n165 = Select(t="", s=w243, f=w232) -> (s? t:f=w245:string)
        n166 = call "Add State to Queue.vi"("State(s) In Front (\"\")"=w245, "State(s) In (\"\")"=w257) -> ("States Out"=w256:string)  [unwired: 13 in]
      }
      frame "获取平行样测试数据" {
        n167 = call "启动日志.vi"("日志信息"=w285, "Slave ID"=w296) -> ()  [unwired: 9 in, 1 out]
        n168 = property class="Clust (严格)"(reference=w283) -> (reference out=w307:refnum<vi>, "Value"=w306:T14)  [unwired: 1 in, 1 out]
        n169 = case shown="\"CODCr\"" w296 {
          tunnel: [sgl 0.0 ("水样实测值") w317 w321 w325 w329 w333] -> w304
          tunnel: [timestamp(0 s since 1904-01-01) ("加标回收数据时间") w316 w320 w324 w328 w332] -> w282
          frame "null", Default {
          }
          frame "氨氮" {
            w314 = u16 3 items=["总磷"=1, "总氮"=2, "氨氮"=3, "CODMn"=21, "CODcr"=22] ("站号")
            n170 = call-poly "获取测试数据.vi"("站号"=w314) -> ("测量数据区"=w315:T15)  [unwired: 10 in]
            n171 = Unbundle By Name(w315) -> ("水样数据时间"=w316:timestamp, "水样实测值"=w317:sgl)
          }
          frame "总磷" {
            w318 = u16 1 items=["总磷"=1, "总氮"=2, "氨氮"=3, "CODMn"=21, "CODcr"=22] ("站号")
            n172 = call-poly "获取测试数据.vi"("站号"=w318) -> ("测量数据区"=w319:T15)  [unwired: 10 in]
            n173 = Unbundle By Name(w319) -> ("水样数据时间"=w320:timestamp, "水样实测值"=w321:sgl)
          }
          frame "总氮" {
            w322 = u16 2 items=["总磷"=1, "总氮"=2, "氨氮"=3, "CODMn"=21, "CODcr"=22] ("站号")
            n174 = call-poly "获取测试数据.vi"("站号"=w322) -> ("测量数据区"=w323:T15)  [unwired: 10 in]
            n175 = Unbundle By Name(w323) -> ("水样数据时间"=w324:timestamp, "水样实测值"=w325:sgl)
          }
          frame "CODMn" {
            w326 = u16 21 items=["总磷"=1, "总氮"=2, "氨氮"=3, "CODMn"=21, "CODcr"=22] ("站号")
            n176 = call-poly "获取测试数据.vi"("站号"=w326) -> ("测量数据区"=w327:T15)  [unwired: 10 in]
            n177 = Unbundle By Name(w327) -> ("水样数据时间"=w328:timestamp, "水样实测值"=w329:sgl)
          }
          frame "CODCr" {
            w330 = u16 22 items=["总磷"=1, "总氮"=2, "氨氮"=3, "CODMn"=21, "CODcr"=22] ("站号")
            n178 = call-poly "获取测试数据.vi"("站号"=w330) -> ("测量数据区"=w331:T15)  [unwired: 10 in]
            n179 = Unbundle By Name(w331) -> ("水样数据时间"=w332:timestamp, "水样实测值"=w333:sgl)
          }
        }
        n180 = Index Array(array=w287, index=10 ("索引")) -> (element=w295:refnum<vi>)
        n181 = property class="DigNum (严格)"(reference=w295) -> (reference out=w293:refnum<vi>, "Value"=w292:u16)  [unwired: 1 in, 1 out]
        n182 = Increment(x=w292) -> (x+1=w291:u16)
        n183 = property class="DigNum (严格)"(reference=w293, "Value"=w291) -> ()  [unwired: 1 in, 2 out]
        n184 = Less Or Equal?(x=w291, y=u16 5) -> (x <= y?=w289:bool)
        n185 = Select(t=w285, s=w289, f="exit") -> (s? t:f=w286:string)
        n186 = Bundle By Name(cluster=w306, "第二次水样测试时间"=w282, "第二次水样浓度值"=w304) -> (w305:T14)
        n187 = local read "平行样启动时间"() -> (w302:timestamp)
        n188 = Subtract(x=w282, y=w302) -> (x-y=w301:dbl)
        n189 = property class="Clust (严格)"(reference=w307, "Value"=w305) -> ()  [unwired: 1 in, 2 out]
        n190 = Absolute Value(x=w301) -> (abs(x)=w298:dbl)
        n191 = Less?(x=w298, y=300.0) -> (x < y?=w297:bool)
        n192 = case shown="假" w297 {
          tunnel: w296 -> [w311 _]
          frame False {
            w310 = "获取平行样数据异常" ("日志信息")
            n193 = call "启动日志.vi"("日志信息"=w310, "Slave ID"=w311) -> ()  [unwired: 9 in, 1 out]
            n194 = call "报警信息记录.vi"("报警信息"=w310, "Slave ID"=w311) -> ()  [unwired: 9 in, 1 out]
          }
          frame True {
          }
        }
        n195 = Select(t="", s=w297, f=w286) -> (s? t:f=w299:string)
        n196 = call "Add State to Queue.vi"("State(s) In Front (\"\")"=w299, "State(s) In (\"\")"=w309) -> ("States Out"=w308:string)  [unwired: 13 in]
      }
      frame "计算加标体积" {
        n197 = call "启动日志.vi"("日志信息"=w336, "Slave ID"=w335) -> ()  [unwired: 9 in, 1 out]
        n198 = property class="Clust (严格)"(reference=w342) -> (reference out=w341:refnum<vi>, "Value"=w340:T4)  [unwired: 1 in, 1 out]
        n199 = call "加标回收率计算.vi"("参数"=w340) -> ("参数 out"=w339:T4)  [unwired: 9 in, 1 out]
        n200 = Bundle By Name(cluster=w339, "加标回收率"=0.0) -> (w338:T4)
        n201 = property class="Clust (严格)"(reference=w341, "Value"=w338) -> ()  [unwired: 1 in, 2 out]
        n202 = call "Add State to Queue.vi"("State(s) In (\"\")"=w344) -> ("States Out"=w343:string)  [unwired: 14 in]
      }
      frame "计算加标回收率" {
        n203 = call "启动日志.vi"("日志信息"=w346, "Slave ID"=w347) -> ()  [unwired: 9 in, 1 out]
        n204 = property class="Clust (严格)"(reference=w351) -> (reference out=w350:refnum<vi>, "Value"=w349:T4)  [unwired: 1 in, 1 out]
        n205 = call "加标回收率计算.vi"("参数"=w349) -> ("参数 out"=w348:T4)  [unwired: 9 in, 1 out]
        n206 = property class="Clust (严格)"(reference=w350, "Value"=w348) -> ()  [unwired: 1 in, 2 out]
        n207 = call "Add State to Queue.vi"("State(s) In (\"\")"=w353) -> ("States Out"=w352:string)  [unwired: 14 in]
      }
      frame "存储加标回收测试数据" {
        n208 = call "启动日志.vi"("日志信息"=w357, "Slave ID"=w358) -> ()  [unwired: 9 in, 1 out]
        n209 = case shown="\"总氮\"" w358 {
          tunnel: ["" "氨氮加标回收率" "总磷加标回收率" "总氮加标回收率" "CODMn加标回收率" "CODCr加标回收率"] -> w359
          frame "null", Default {
          }
          frame "氨氮" {
          }
          frame "总磷" {
          }
          frame "总氮" {
          }
          frame "CODMn" {
          }
          frame "CODCr" {
          }
        }
        n210 = property class="Clust (严格)"(reference=w369) -> ("Value"=w366:T4)  [unwired: 1 in, 2 out]
        n211 = Unbundle By Name(w366) -> ("加标前水样浓度"=w365:dbl, "加标后水样浓度"=w364:dbl, "加标母液浓度"=w363:dbl, "加标体积"=w362:dbl, "加标水杯定容体积"=w361:dbl, "加标回收率"=w360:dbl)
        n212 = call "Add State to Queue.vi"("State(s) In (\"\")"=w371) -> ("States Out"=w370:string)  [unwired: 14 in]
        n213 = Bundle By Name(cluster=T7 {"时间"=timestamp(0 s since 1904-01-01), "参数"="", "数据类型"="N", "加标回收率"=0.0, "加标前水样测试时间"=timestamp(0 s since 1904-01-01), "加标前水样浓度值"=0.0, "加标后水样浓度值"=0.0, "加标母液浓度值"=0.0, "加标体积"=0.0, "加标水杯定容体积"=0.0} ("data in"), "时间"="加标回收测试时间", "参数"=w359, "加标前水样测试时间"="水样测试时间", "加标前水样浓度值"=w365, "加标后水样浓度值"=w364, "加标母液浓度值"=w363, "加标体积"=w362, "加标水杯定容体积"=w361, "加标回收率"=w360) -> (w355:T7)
        n214 = call "加标回收数据插入.vi"("data in"=w355) -> ()  [unwired: 10 in, 1 out]
      }
      frame "存储平行样测试数据" {
        n215 = call "启动日志.vi"("日志信息"=w384, "Slave ID"=w385) -> ()  [unwired: 9 in, 1 out]
        n216 = property class="Clust (严格)"(reference=w382) -> (reference out=w380:refnum<vi>, "Value"=w381:T14)  [unwired: 1 in, 1 out]
        n217 = case shown="\"CODMn\"" w385 {
          tunnel: ["" "氨氮" "总磷" "总氮" "CODMn" "CODCr"] -> w378
          frame "null", Default {
          }
          frame "氨氮" {
          }
          frame "总磷" {
          }
          frame "总氮" {
          }
          frame "CODMn" {
          }
          frame "CODCr" {
          }
        }
        n218 = call "Add State to Queue.vi"("State(s) In (\"\")"=w387) -> ("States Out"=w386:string)  [unwired: 14 in]
        n219 = Bundle By Name(cluster=w381, "参数"=w378) -> (w379:T14)
        n220 = property class="Clust (严格)"(reference=w380, "Value"=w379) -> ()  [unwired: 1 in, 2 out]
        n221 = call "平行样数据插入.vi"("平行样测试数据"=w379) -> ()  [unwired: 10 in, 1 out]
      }
      frame "存储集成干预测试数据" {
        n222 = call "启动日志.vi"("日志信息"=w401, "Slave ID"=w396) -> ()  [unwired: 9 in, 1 out]
        n223 = property class="Clust (严格)"(reference=w399) -> (reference out=w397:refnum<vi>, "Value"=w398:T2)  [unwired: 1 in, 1 out]
        n224 = case shown="\"CODMn\"" w396 {
          tunnel: ["" "氨氮" "总磷" "总氮" "CODMn" "CODCr"] -> w395
          frame "null", Default {
          }
          frame "氨氮" {
          }
          frame "总磷" {
          }
          frame "总氮" {
          }
          frame "CODMn" {
          }
          frame "CODCr" {
          }
        }
        n225 = call "Add State to Queue.vi"("State(s) In (\"\")"=w403) -> ("States Out"=w402:string)  [unwired: 14 in]
        n226 = Bundle By Name(cluster=w398, "参数"=w395) -> (w394:T2)
        n227 = property class="Clust (严格)"(reference=w397, "Value"=w394) -> ()  [unwired: 1 in, 2 out]
        n228 = call "集成干预数据插入.vi"("集成干预测试数据"=w394) -> ()  [unwired: 10 in, 1 out]
      }
      frame "流程结束" {
        n229 = global read "ZK非断电保存全局变量.vi" "流程运行状态标记位"() -> (w416:T6)
        n230 = case shown="\"CODCr\"" w414 {
          tunnel: "空闲" -> [_ w420 w421 w422 w423 w424]
          frame "null", Default {
          }
          frame "氨氮" {
            n231 = global write "ZK非断电保存全局变量.vi" "氨氮加标模块运行状态"(w420) -> ()
          }
          frame "总磷" {
            n232 = global write "ZK非断电保存全局变量.vi" "总磷加标模块运行状态"(w421) -> ()
          }
          frame "总氮" {
            n233 = global write "ZK非断电保存全局变量.vi" "总氮加标模块运行状态"(w422) -> ()
          }
          frame "CODMn" {
            n234 = global write "ZK非断电保存全局变量.vi" "CODMn加标模块运行状态"(w423) -> ()
          }
          frame "CODCr" {
            n235 = global write "ZK非断电保存全局变量.vi" "CODcr加标模块运行状态"(w424) -> ()
          }
        }
        n236 = Concatenate Strings("----->>" ("字符串"), w413) -> (w412:string)
        n237 = case shown="\"总磷\"" w414 {
          tunnel: w416 -> [_ w427 w428 w431 w434 w437]
          frame "null", Default {
          }
          frame "氨氮" {
            n238 = Bundle By Name(cluster=w427, "氨氮"=FALSE) -> (w426:T6)
            n239 = global write "ZK非断电保存全局变量.vi" "流程运行状态标记位"(w426) -> ()
          }
          frame "总磷" {
            n240 = Bundle By Name(cluster=w428, "总磷"=FALSE ("氨氮")) -> (w430:T6)
            n241 = global write "ZK非断电保存全局变量.vi" "流程运行状态标记位"(w430) -> ()
          }
          frame "总氮" {
            n242 = Bundle By Name(cluster=w431, "总氮"=FALSE ("氨氮")) -> (w433:T6)
            n243 = global write "ZK非断电保存全局变量.vi" "流程运行状态标记位"(w433) -> ()
          }
          frame "CODMn" {
            n244 = Bundle By Name(cluster=w434, "CODMn"=FALSE ("氨氮")) -> (w436:T6)
            n245 = global write "ZK非断电保存全局变量.vi" "流程运行状态标记位"(w436) -> ()
          }
          frame "CODCr" {
            n246 = Bundle By Name(cluster=w437, "CODCr"=FALSE ("氨氮")) -> (w439:T6)
            n247 = global write "ZK非断电保存全局变量.vi" "流程运行状态标记位"(w439) -> ()
          }
        }
        n248 = call "启动日志.vi"("日志信息"=w412, "Slave ID"=w414) -> ()  [unwired: 9 in, 1 out]
        n249 = call "Add State to Queue.vi"("State(s) In (\"\")"=w419) -> ("States Out"=w418:string)  [unwired: 14 in]
      }
      frame "流程退出" {
        n250 = Concatenate Strings("----->>" ("字符串"), w443) -> (w442:string)
        n251 = call "启动日志.vi"("日志信息"=w442, "Slave ID"=w444) -> ()  [unwired: 9 in, 1 out]
        n252 = call "Add State to Queue.vi"("State(s) In (\"\")"=w447) -> ("States Out"=w446:string)  [unwired: 14 in]
      }
      frame "-------------------# 采配水流程 #-------------------" {
        n253 = call "Add State to Queue.vi"("State(s) In (\"\")"=w450) -> ("States Out"=w449:string)  [unwired: 14 in]
      }
      frame "采水单元启动水样测试流程" {
        n254 = call "启动日志.vi"("日志信息"=w453, "Slave ID"=w454) -> ()  [unwired: 9 in, 1 out]
        n255 = call "采配水启动器.vi"("启动/停止命令"=T8."水样测试（全流程）") -> ()  [unwired: 10 in, 1 out]
        n256 = Index Array(array=w459) -> (element=w458:refnum<vi>)  [unwired: 1 in]
        n257 = property class="DigNum (严格)"(reference=w458) -> (reference out=w457:refnum<vi>, "Value"=w456:u16)  [unwired: 1 in, 1 out]
        n258 = Increment(x=w456) -> (x+1=w455:u16)
        n259 = property class="DigNum (严格)"(reference=w457, "Value"=w455) -> ()  [unwired: 1 in, 2 out]
        n260 = call "Add State to Queue.vi"("State(s) In (\"\")"=w461) -> ("States Out"=w460:string)  [unwired: 14 in]
      }
      frame "采水单元启动加标回收流程" {
        n261 = call "启动日志.vi"("日志信息"=w464, "Slave ID"=w465) -> ()  [unwired: 9 in, 1 out]
        n262 = call "采配水启动器.vi"("启动/停止命令"=T8."加标回收") -> ()  [unwired: 10 in, 1 out]
        n263 = Index Array(array=w470) -> (element=w469:refnum<vi>)  [unwired: 1 in]
        n264 = property class="DigNum (严格)"(reference=w469) -> (reference out=w468:refnum<vi>, "Value"=w467:u16)  [unwired: 1 in, 1 out]
        n265 = Increment(x=w467) -> (x+1=w466:u16)
        n266 = property class="DigNum (严格)"(reference=w468, "Value"=w466) -> ()  [unwired: 1 in, 2 out]
        n267 = call "Add State to Queue.vi"("State(s) In (\"\")"=w472) -> ("States Out"=w471:string)  [unwired: 14 in]
      }
      frame "判断采水单元水样测试流程是否启动" {
        n268 = call "启动日志.vi"("日志信息"=w476, "Slave ID"=w475) -> ()  [unwired: 9 in, 1 out]
        n269 = call "获取采配水运行状态.vi"() -> ("运行流程"=w489:T10)  [unwired: 10 in, 1 out]
        n270 = Equal?(x=T9."待机" ("运行流程"), y=w489) -> (x = y?=w488:bool)
        n271 = Index Array(array=w480, index=0 ("索引")) -> (element=w479:refnum<vi>)
        n272 = property class="DigNum (严格)"(reference=w479) -> ("Value"=w478:u16)  [unwired: 1 in, 2 out]
        n273 = Greater Or Equal?(x=w478, y=u16 5) -> (x >= y?=w474:bool)
        n274 = Select(t="采水单元启动水样测试流程\n判断采水单元水样测试流程是否启动" ("State(s) In (\"\")"), s=w488, f="") -> (s? t:f=w483:string)
        n275 = case shown="真" w474 {
          tunnel: w475 -> [_ w493]
          frame False {
          }
          frame True {
            w492 = "采水单元启动失败" ("日志信息")
            n276 = call "启动日志.vi"("日志信息"=w492, "Slave ID"=w493) -> ()  [unwired: 9 in, 1 out]
            n277 = call "报警信息记录.vi"("报警信息"=w492, "Slave ID"=w493) -> ()  [unwired: 9 in, 1 out]
          }
        }
        n278 = Select(t="流程结束" ("State(s) In (\"\")"), s=w474, f=w483) -> (s? t:f=w482:string)
        n279 = call "Add State to Queue.vi"("State(s) In Front (\"\")"=w482, "State(s) In (\"\")"=w491) -> ("States Out"=w490:string)  [unwired: 13 in]
      }
      frame "判断采水单元加标回收流程是否启动" {
        n280 = call "启动日志.vi"("日志信息"=w497, "Slave ID"=w496) -> ()  [unwired: 9 in, 1 out]
        n281 = call "获取采配水运行状态.vi"() -> ("运行流程"=w511:T10)  [unwired: 10 in, 1 out]
        n282 = Equal?(x=T9."待机" ("运行流程"), y=w511) -> (x = y?=w510:bool)
        n283 = Index Array(array=w502, index=0 ("索引")) -> (element=w501:refnum<vi>)
        n284 = property class="DigNum (严格)"(reference=w501) -> ("Value"=w500:u16)  [unwired: 1 in, 2 out]
        n285 = Greater Or Equal?(x=w500, y=u16 5) -> (x >= y?=w495:bool)
        n286 = Select(t="采水单元启动加标回收流程\n判断采水单元加标回收流程是否启动" ("State(s) In (\"\")"), s=w510, f="") -> (s? t:f=w505:string)
        n287 = case shown="真" w495 {
          tunnel: w496 -> [_ w514]
          frame False {
          }
          frame True {
            w513 = "采水单元启动失败" ("日志信息")
            n288 = call "启动日志.vi"("日志信息"=w513, "Slave ID"=w514) -> ()  [unwired: 9 in, 1 out]
            n289 = call "报警信息记录.vi"("报警信息"=w513, "Slave ID"=w514) -> ()  [unwired: 9 in, 1 out]
          }
        }
        n290 = Select(t="流程结束" ("State(s) In (\"\")"), s=w495, f=w505) -> (s? t:f=w504:string)
        n291 = call "Add State to Queue.vi"("State(s) In Front (\"\")"=w504, "State(s) In (\"\")"=w498) -> ("States Out"=w512:string)  [unwired: 13 in]
      }
      frame "采水单元润洗" {
        n292 = call "获取采配水运行状态.vi"() -> ("运行流程"=w525:T10)  [unwired: 10 in, 1 out]
        n293 = Equal To 0?(x=w525) -> (x = 0?=w517:bool)
        n294 = Less?(x=w525, y=T9."采样" ("运行流程")) -> (x < y?=w528:bool)
        n295 = Greater?(x=w525, y=T9."待机" ("运行流程")) -> (0:w529:bool)
        n296 = case shown="真" w515 {
          tunnel: w518 -> [_ w535]
          tunnel: w519 -> [_ w534]
          frame False {
          }
          frame True {
            n297 = call "启动日志.vi"("日志信息"=w534, "Slave ID"=w535) -> ()  [unwired: 9 in, 1 out]
          }
        }
        n298 = And(x=w528, y=w529) -> (x .and. y?=w527:bool)
        n299 = case shown="真" w517 {
          tunnel: w518 -> [_ w533]
          frame False {
          }
          frame True {
            w532 = "采水单元流程中断" ("日志信息")
            n300 = call "启动日志.vi"("日志信息"=w532, "Slave ID"=w533) -> ()  [unwired: 9 in, 1 out]
            n301 = call "报警信息记录.vi"("报警信息"=w532, "Slave ID"=w533) -> ()  [unwired: 9 in, 1 out]
          }
        }
        n302 = Select(t=w519, s=w527, f="") -> (s? t:f=w523:string)
        n303 = Select(t="流程结束" ("State(s) In (\"\")"), s=w517, f=w523) -> (s? t:f=w522:string)
        n304 = call "Add State to Queue.vi"("State(s) In Front (\"\")"=w522, "State(s) In (\"\")"=w531) -> ("States Out"=w530:string)  [unwired: 13 in]
      }
      frame "采水单元采样" {
        n305 = call "获取采配水运行状态.vi"() -> ("运行流程"=w542:T10)  [unwired: 10 in, 1 out]
        n306 = Equal To 0?(x=w542) -> (x = 0?=w539:bool)
        n307 = Equal?(x=T9."采样" ("运行流程"), y=w542) -> (x = y?=w541:bool)
        n308 = case shown="真" w536 {
          tunnel: w538 -> [_ w553]
          tunnel: w540 -> [_ w552]
          frame False {
          }
          frame True {
            n309 = call "启动日志.vi"("日志信息"=w552, "Slave ID"=w553) -> ()  [unwired: 9 in, 1 out]
          }
        }
        n310 = case shown="真" w539 {
          tunnel: w538 -> [_ w551]
          frame False {
          }
          frame True {
            w550 = "采水单元流程中断" ("日志信息")
            n311 = call "启动日志.vi"("日志信息"=w550, "Slave ID"=w551) -> ()  [unwired: 9 in, 1 out]
            n312 = call "报警信息记录.vi"("报警信息"=w550, "Slave ID"=w551) -> ()  [unwired: 9 in, 1 out]
          }
        }
        n313 = Select(t=w540, s=w541, f="") -> (s? t:f=w545:string)
        n314 = Select(t="流程结束" ("State(s) In (\"\")"), s=w539, f=w545) -> (s? t:f=w544:string)
        n315 = call "Add State to Queue.vi"("State(s) In Front (\"\")"=w544, "State(s) In (\"\")"=w549) -> ("States Out"=w548:string)  [unwired: 13 in]
      }
      frame "水样沉淀" {
        n316 = global read "系统交互.vi" "站点类型"() -> (w559:enum16{"一体站", "固定站", "浮船", "一体站V1-V3"})
        n317 = case shown="真" w555 {
          tunnel: w558 -> [_ w577]
          tunnel: w561 -> [_ w576]
          frame False {
          }
          frame True {
            n318 = call "启动日志.vi"("日志信息"=w576, "Slave ID"=w577) -> ()  [unwired: 9 in, 1 out]
          }
        }
        n319 = case shown="\"浮船\"" w559 {
          tunnel: [w573 _ _] -> w560
          tunnel: w555 -> [w572 _ _]
          frame "一体站", Default {
            n320 = case shown="真" w572 {
              tunnel: [_ w574] -> w573
              frame False {
              }
              frame True {
                n321 = call "质控模块润洗OK命令.vi"("质控润洗OK"=TRUE) -> ("error out"=w574:errorcluster)  [unwired: 10 in]
              }
            }
          }
          frame "固定站" {
          }
          frame "浮船" {
          }
        }
        n322 = call "获取采配水运行状态.vi"("error in (no error)"=w560) -> ("运行流程"=w565:T10)  [unwired: 9 in, 1 out]
        n323 = Equal To 0?(x=w565) -> (x = 0?=w557:bool)
        n324 = Equal?(x=采配水通用流程."沉淀" ("运行流程"), y=w565) -> (x = y?=w567:bool)
        n325 = case shown="真" w557 {
          tunnel: w558 -> [_ w571]
          frame False {
          }
          frame True {
            w570 = "采水单元流程中断" ("日志信息")
            n326 = call "启动日志.vi"("日志信息"=w570, "Slave ID"=w571) -> ()  [unwired: 9 in, 1 out]
            n327 = call "报警信息记录.vi"("报警信息"=w570, "Slave ID"=w571) -> ()  [unwired: 9 in, 1 out]
          }
        }
        n328 = Select(t=w561, s=w567, f="") -> (s? t:f=w563:string)
        n329 = Select(t="流程结束" ("State(s) In (\"\")"), s=w557, f=w563) -> (s? t:f=w562:string)
        n330 = call "Add State to Queue.vi"("State(s) In Front (\"\")"=w562, "State(s) In (\"\")"=w569) -> ("States Out"=w568:string)  [unwired: 13 in]
      }
      frame "水样配水" {
        n331 = call "获取采配水运行状态.vi"() -> ("运行流程"=w588:T10)  [unwired: 10 in, 1 out]
        n332 = Equal To 0?(x=w588) -> (x = 0?=w582:bool)
        n333 = Equal?(x=采配水通用流程."配水" ("运行流程"), y=w588) -> (x = y?=w589:bool)
        n334 = case shown="真" w579 {
          tunnel: w581 -> [_ w595]
          tunnel: w583 -> [_ w594]
          frame False {
          }
          frame True {
            n335 = call "启动日志.vi"("日志信息"=w594, "Slave ID"=w595) -> ()  [unwired: 9 in, 1 out]
          }
        }
        n336 = case shown="真" w582 {
          tunnel: w581 -> [_ w593]
          frame False {
          }
          frame True {
            w592 = "采水单元流程中断" ("日志信息")
            n337 = call "启动日志.vi"("日志信息"=w592, "Slave ID"=w593) -> ()  [unwired: 9 in, 1 out]
            n338 = call "报警信息记录.vi"("报警信息"=w592, "Slave ID"=w593) -> ()  [unwired: 9 in, 1 out]
          }
        }
        n339 = Select(t="", s=w589, f=w583) -> (s? t:f=w586:string)
        n340 = Select(t="流程结束" ("State(s) In (\"\")"), s=w582, f=w586) -> (s? t:f=w585:string)
        n341 = call "Add State to Queue.vi"("State(s) In Front (\"\")"=w585, "State(s) In (\"\")"=w591) -> ("States Out"=w590:string)  [unwired: 13 in]
      }
      frame "-------------------# 质控模块流程 #-------------------" {
        n342 = call "Add State to Queue.vi"("State(s) In (\"\")"=w598) -> ("States Out"=w597:string)  [unwired: 14 in]
      }
      frame "质控单元启动采样" {
        n343 = call "启动日志.vi"("日志信息"=w600, "Slave ID"=w601) -> ()  [unwired: 9 in, 1 out]
        n344 = call "ZK流程控制.vi"("流程控制"=质控流程控制."启动进样流程", "Slave ID"=w601) -> ()  [unwired: 9 in, 1 out]
        n345 = Index Array(array=w603, index=2 ("索引")) -> (element=w607:refnum<vi>)
        n346 = property class="DigNum (严格)"(reference=w607) -> (reference out=w606:refnum<vi>, "Value"=w605:u16)  [unwired: 1 in, 1 out]
        n347 = Increment(x=w605) -> (x+1=w604:u16)
        n348 = property class="DigNum (严格)"(reference=w606, "Value"=w604) -> ()  [unwired: 1 in, 2 out]
        n349 = call "Add State to Queue.vi"("State(s) In (\"\")"=w610) -> ("States Out"=w609:string)  [unwired: 14 in]
      }
      frame "质控单元写入加标体积" {
        n350 = call "启动日志.vi"("日志信息"=w618, "Slave ID"=w612) -> ()  [unwired: 9 in, 1 out]
        n351 = property class="Clust (严格)"(reference=w623) -> ("Value"=w622:T4)  [unwired: 1 in, 2 out]
        n352 = Index Array(array=w617, index=8 ("索引")) -> (element=w615:refnum<vi>)
        n353 = Unbundle By Name(w622) -> ("加标体积"=w621:dbl)
        n354 = property class="DigNum (严格)"(reference=w615) -> (reference out=w613:refnum<vi>, "Value"=w614:u16)  [unwired: 1 in, 1 out]
        n355 = call "ZK加标体积写入.vi"("加标体积"=w621, "Slave ID"=w612) -> ("error out"=w620:errorcluster)  [unwired: 9 in]
        n356 = case shown="错误" w620 {
          tunnel: [_ w628] -> w619
          tunnel: w618 -> [_ w630]
          tunnel: w614 -> [_ w632]
          tunnel: w613 -> [_ w634]
          tunnel: w612 -> [_ w626]
          frame No Error {
          }
          frame Error {
            n357 = Increment(x=w632) -> (x+1=w633:u16)
            n358 = Greater Or Equal?(x=w632, y=u16 5) -> (x >= y?=w627:bool)
            n359 = property class="DigNum (严格)"(reference=w634, "Value"=w633) -> ()  [unwired: 1 in, 2 out]
            n360 = case shown="真" w627 {
              tunnel: w626 -> [_ w636]
              frame False {
              }
              frame True {
                w635 = "加标体积写入异常" ("报警信息")
                n361 = call "启动日志.vi"("日志信息"=w635, "Slave ID"=w636) -> ()  [unwired: 9 in, 1 out]
                n362 = call "报警信息记录.vi"("报警信息"=w635, "Slave ID"=w636) -> ()  [unwired: 9 in, 1 out]
              }
            }
            n363 = Select(t="流程结束", s=w627, f=w630) -> (s? t:f=w628:string)
          }
        }
        n364 = call "Add State to Queue.vi"("State(s) In Front (\"\")"=w619, "State(s) In (\"\")"=w625) -> ("States Out"=w624:string)  [unwired: 13 in]
      }
      frame "质控单元启动加标" {
        n365 = call "启动日志.vi"("日志信息"=w638, "Slave ID"=w639) -> ()  [unwired: 9 in, 1 out]
        n366 = call "ZK流程控制.vi"("流程控制"=质控流程控制."启动加标流程", "Slave ID"=w639) -> ()  [unwired: 9 in, 1 out]
        n367 = Index Array(array=w642, index=3 ("索引")) -> (element=w641:refnum<vi>)
        n368 = property class="DigNum (严格)"(reference=w641) -> (reference out=w645:refnum<vi>, "Value"=w644:u16)  [unwired: 1 in, 1 out]
        n369 = Increment(x=w644) -> (x+1=w643:u16)
        n370 = property class="DigNum (严格)"(reference=w645, "Value"=w643) -> ()  [unwired: 1 in, 2 out]
        n371 = call "Add State to Queue.vi"("State(s) In (\"\")"=w648) -> ("States Out"=w647:string)  [unwired: 14 in]
      }
      frame "质控单元启动排液" {
        n372 = call "启动日志.vi"("日志信息"=w650, "Slave ID"=w651) -> ()  [unwired: 9 in, 1 out]
        n373 = call "ZK流程控制.vi"("流程控制"=质控流程控制."启动排液流程", "Slave ID"=w651) -> ()  [unwired: 9 in, 1 out]
        n374 = Index Array(array=w654, index=4 ("索引")) -> (element=w653:refnum<vi>)
        n375 = property class="DigNum (严格)"(reference=w653) -> (reference out=w657:refnum<vi>, "Value"=w656:u16)  [unwired: 1 in, 1 out]
        n376 = Increment(x=w656) -> (x+1=w655:u16)
        n377 = property class="DigNum (严格)"(reference=w657, "Value"=w655) -> ()  [unwired: 1 in, 2 out]
        n378 = call "Add State to Queue.vi"("State(s) In (\"\")"=w660) -> ("States Out"=w659:string)  [unwired: 14 in]
      }
      frame "判断质控单元采样是否启动成功" {
        n379 = case shown="真" w668 {
          tunnel: w662 -> [_ w686]
          tunnel: w669 -> [_ w685]
          frame False {
          }
          frame True {
            n380 = call "启动日志.vi"("日志信息"=w686, "Slave ID"=w685) -> ()  [unwired: 9 in, 1 out]
          }
        }
        n381 = case shown="\"CODCr\"" w669 {
          tunnel: [T12."待机" ("运行状态") w690 w692 w694 w696 w698] -> w681
          frame "null", Default {
          }
          frame "氨氮" {
            n382 = global read "ZK非断电保存全局变量.vi" "氨氮质控仪器状态"() -> (w691:T17)
            n383 = Unbundle By Name(w691) -> ("运行状态"=w690:T18)
          }
          frame "总磷" {
            n384 = global read "ZK非断电保存全局变量.vi" "总磷质控仪器状态"() -> (w693:T17)
            n385 = Unbundle By Name(w693) -> ("运行状态"=w692:T18)
          }
          frame "总氮" {
            n386 = global read "ZK非断电保存全局变量.vi" "总氮质控仪器状态"() -> (w695:T17)
            n387 = Unbundle By Name(w695) -> ("运行状态"=w694:T18)
          }
          frame "CODMn" {
            n388 = global read "ZK非断电保存全局变量.vi" "CODMn质控仪器状态"() -> (w697:T17)
            n389 = Unbundle By Name(w697) -> ("运行状态"=w696:T18)
          }
          frame "CODCr" {
            n390 = global read "ZK非断电保存全局变量.vi" "CODCr质控仪器状态"() -> (w699:T17)
            n391 = Unbundle By Name(w699) -> ("运行状态"=w698:T18)
          }
        }
        n392 = Index Array(array=w674, index=2 ("索引")) -> (element=w673:refnum<vi>)
        n393 = Greater Or Equal?(x=w667, y=10) -> (x >= y?=w664:bool)
        n394 = property class="DigNum (严格)"(reference=w673) -> ("Value"=w672:u16)  [unwired: 1 in, 2 out]
        n395 = Select(t="质控单元启动采样\n判断质控单元采样是否启动成功" ("State(s) In (\"\")"), s=w664, f=w662) -> (s? t:f=w661:string)
        n396 = Greater Or Equal?(x=w672, y=u16 5) -> (x >= y?=w670:bool)
        n397 = case shown="真" w670 {
          tunnel: w669 -> [_ w688]
          frame False {
          }
          frame True {
            w687 = "质控单元采样启动失败" ("日志信息")
            n398 = call "启动日志.vi"("日志信息"=w687, "Slave ID"=w688) -> ()  [unwired: 9 in, 1 out]
            n399 = call "报警信息记录.vi"("报警信息"=w687, "Slave ID"=w688) -> ()  [unwired: 9 in, 1 out]
          }
        }
        n400 = Not Equal?(x=w681, y=T12."待机") -> (x != y?=w680:bool)
        n401 = And(x=w664, y=w680) -> (x .and. y?=w665:bool)
        n402 = Select(t="", s=w665, f=w661) -> (s? t:f=w678:string)
        n403 = Select(t="流程结束" ("State(s) In (\"\")"), s=w670, f=w678) -> (s? t:f=w676:string)
        n404 = call "Add State to Queue.vi"("State(s) In Front (\"\")"=w676, "State(s) In (\"\")"=w684) -> ("States Out"=w683:string)  [unwired: 13 in]
      }
      frame "判断质控单元加标是否启动成功" {
        n405 = case shown="真" w706 {
          tunnel: w701 -> [_ w725]
          tunnel: w708 -> [_ w724]
          frame False {
          }
          frame True {
            n406 = call "启动日志.vi"("日志信息"=w725, "Slave ID"=w724) -> ()  [unwired: 9 in, 1 out]
          }
        }
        n407 = case shown="\"CODCr\"" w708 {
          tunnel: [T12."异常停机" ("运行状态") w729 w731 w733 w735 w737] -> w720
          frame "null", Default {
          }
          frame "氨氮" {
            n408 = global read "ZK非断电保存全局变量.vi" "氨氮质控仪器状态"() -> (w730:T17)
            n409 = Unbundle By Name(w730) -> ("运行状态"=w729:T18)
          }
          frame "总磷" {
            n410 = global read "ZK非断电保存全局变量.vi" "总磷质控仪器状态"() -> (w732:T17)
            n411 = Unbundle By Name(w732) -> ("运行状态"=w731:T18)
          }
          frame "总氮" {
            n412 = global read "ZK非断电保存全局变量.vi" "总氮质控仪器状态"() -> (w734:T17)
            n413 = Unbundle By Name(w734) -> ("运行状态"=w733:T18)
          }
          frame "CODMn" {
            n414 = global read "ZK非断电保存全局变量.vi" "CODMn质控仪器状态"() -> (w736:T17)
            n415 = Unbundle By Name(w736) -> ("运行状态"=w735:T18)
          }
          frame "CODCr" {
            n416 = global read "ZK非断电保存全局变量.vi" "CODCr质控仪器状态"() -> (w738:T17)
            n417 = Unbundle By Name(w738) -> ("运行状态"=w737:T18)
          }
        }
        n418 = Index Array(array=w713, index=3 ("索引")) -> (element=w712:refnum<vi>)
        n419 = Greater Or Equal?(x=w707, y=10) -> (x >= y?=w703:bool)
        n420 = property class="DigNum (严格)"(reference=w712) -> ("Value"=w711:u16)  [unwired: 1 in, 2 out]
        n421 = Select(t="质控单元启动加标\n判断质控单元加标是否启动成功" ("State(s) In (\"\")"), s=w703, f=w701) -> (s? t:f=w700:string)
        n422 = Greater Or Equal?(x=w711, y=u16 5) -> (x >= y?=w709:bool)
        n423 = case shown="真" w709 {
          tunnel: w708 -> [_ w727]
          frame False {
          }
          frame True {
            w726 = "质控单元加标启动失败" ("日志信息")
            n424 = call "启动日志.vi"("日志信息"=w726, "Slave ID"=w727) -> ()  [unwired: 9 in, 1 out]
            n425 = call "报警信息记录.vi"("报警信息"=w726, "Slave ID"=w727) -> ()  [unwired: 9 in, 1 out]
          }
        }
        n426 = Not Equal?(x=w720, y=T12."待机") -> (x != y?=w719:bool)
        n427 = And(x=w703, y=w719) -> (x .and. y?=w704:bool)
        n428 = Select(t="", s=w704, f=w700) -> (s? t:f=w717:string)
        n429 = Select(t="流程结束" ("State(s) In (\"\")"), s=w709, f=w717) -> (s? t:f=w715:string)
        n430 = call "Add State to Queue.vi"("State(s) In Front (\"\")"=w715, "State(s) In (\"\")"=w723) -> ("States Out"=w722:string)  [unwired: 13 in]
      }
      frame "判断质控单元排液是否启动成功" {
        n431 = case shown="真" w746 {
          tunnel: w740 -> [_ w764]
          tunnel: w747 -> [_ w763]
          frame False {
          }
          frame True {
            n432 = call "启动日志.vi"("日志信息"=w764, "Slave ID"=w763) -> ()  [unwired: 9 in, 1 out]
          }
        }
        n433 = case shown="\"氨氮\"" w747 {
          tunnel: [T12."异常停机" ("运行状态") w768 w770 w772 w774 w776] -> w759
          frame "null", Default {
          }
          frame "氨氮" {
            n434 = global read "ZK非断电保存全局变量.vi" "氨氮质控仪器状态"() -> (w769:T17)
            n435 = Unbundle By Name(w769) -> ("运行状态"=w768:T18)
          }
          frame "总磷" {
            n436 = global read "ZK非断电保存全局变量.vi" "总磷质控仪器状态"() -> (w771:T17)
            n437 = Unbundle By Name(w771) -> ("运行状态"=w770:T18)
          }
          frame "总氮" {
            n438 = global read "ZK非断电保存全局变量.vi" "总氮质控仪器状态"() -> (w773:T17)
            n439 = Unbundle By Name(w773) -> ("运行状态"=w772:T18)
          }
          frame "CODMn" {
            n440 = global read "ZK非断电保存全局变量.vi" "CODMn质控仪器状态"() -> (w775:T17)
            n441 = Unbundle By Name(w775) -> ("运行状态"=w774:T18)
          }
          frame "CODCr" {
            n442 = global read "ZK非断电保存全局变量.vi" "CODCr质控仪器状态"() -> (w777:T17)
            n443 = Unbundle By Name(w777) -> ("运行状态"=w776:T18)
          }
        }
        n444 = Index Array(array=w752, index=4 ("索引")) -> (element=w751:refnum<vi>)
        n445 = Greater Or Equal?(x=w745, y=10) -> (x >= y?=w742:bool)
        n446 = property class="DigNum (严格)"(reference=w751) -> ("Value"=w750:u16)  [unwired: 1 in, 2 out]
        n447 = Select(t="质控单元启动排液\n判断质控单元排液是否启动成功" ("State(s) In (\"\")"), s=w742, f=w740) -> (s? t:f=w739:string)
        n448 = Greater Or Equal?(x=w750, y=u16 5) -> (x >= y?=w748:bool)
        n449 = case shown="真" w748 {
          tunnel: w747 -> [_ w766]
          frame False {
          }
          frame True {
            w765 = "质控单元排液启动失败" ("日志信息")
            n450 = call "启动日志.vi"("日志信息"=w765, "Slave ID"=w766) -> ()  [unwired: 9 in, 1 out]
            n451 = call "报警信息记录.vi"("报警信息"=w765, "Slave ID"=w766) -> ()  [unwired: 9 in, 1 out]
          }
        }
        n452 = Not Equal?(x=w759, y=T12."等待取样") -> (x != y?=w758:bool)
        n453 = And(x=w742, y=w758) -> (x .and. y?=w743:bool)
        n454 = Select(t="", s=w743, f=w739) -> (s? t:f=w756:string)
        n455 = Select(t="流程结束" ("State(s) In (\"\")"), s=w748, f=w756) -> (s? t:f=w754:string)
        n456 = call "Add State to Queue.vi"("State(s) In Front (\"\")"=w754, "State(s) In (\"\")"=w762) -> ("States Out"=w761:string)  [unwired: 13 in]
      }
      frame "质控单元采样中", "质控单元加标中" {
        n457 = case shown="真" w782 {
          tunnel: w783 -> [_ w802]
          tunnel: w789 -> [_ w801]
          frame False {
          }
          frame True {
            n458 = call "启动日志.vi"("日志信息"=w801, "Slave ID"=w802) -> ()  [unwired: 9 in, 1 out]
          }
        }
        n459 = case shown="\"CODCr\"" w783 {
          tunnel: [T12."待机" ("运行状态") w804 w806 w808 w810 w812] -> w788
          frame "null", Default {
          }
          frame "氨氮" {
            n460 = global read "ZK非断电保存全局变量.vi" "氨氮质控仪器状态"() -> (w805:T17)
            n461 = Unbundle By Name(w805) -> ("运行状态"=w804:T18)
          }
          frame "总磷" {
            n462 = global read "ZK非断电保存全局变量.vi" "总磷质控仪器状态"() -> (w807:T17)
            n463 = Unbundle By Name(w807) -> ("运行状态"=w806:T18)
          }
          frame "总氮" {
            n464 = global read "ZK非断电保存全局变量.vi" "总氮质控仪器状态"() -> (w809:T17)
            n465 = Unbundle By Name(w809) -> ("运行状态"=w808:T18)
          }
          frame "CODMn" {
            n466 = global read "ZK非断电保存全局变量.vi" "CODMn质控仪器状态"() -> (w811:T17)
            n467 = Unbundle By Name(w811) -> ("运行状态"=w810:T18)
          }
          frame "CODCr" {
            n468 = global read "ZK非断电保存全局变量.vi" "CODCr质控仪器状态"() -> (w813:T17)
            n469 = Unbundle By Name(w813) -> ("运行状态"=w812:T18)
          }
        }
        n470 = Greater Or Equal?(x=w781, y=15) -> (x >= y?=w778:bool)
        n471 = Equal?(x=w788, y=T12."异常停机") -> (x = y?=w785:bool)
        n472 = Equal?(x=w788, y=T12."待机") -> (x = y?=w786:bool)
        n473 = Equal?(x=w788, y=T12."等待取样") -> (x = y?=w794:bool)
        n474 = Or(x=w785, y=w786) -> (x .or. y?=w784:bool)
        n475 = And(x=w778, y=w794) -> (x .and. y?=w779:bool)
        n476 = case shown="真" w784 {
          tunnel: w783 -> [_ w800]
          frame False {
          }
          frame True {
            w799 = "质控单元流程中断" ("日志信息")
            n477 = call "启动日志.vi"("日志信息"=w799, "Slave ID"=w800) -> ()  [unwired: 9 in, 1 out]
            n478 = call "报警信息记录.vi"("报警信息"=w799, "Slave ID"=w800) -> ()  [unwired: 9 in, 1 out]
          }
        }
        n479 = Select(t="", s=w779, f=w789) -> (s? t:f=w792:string)
        n480 = Select(t="流程结束" ("State(s) In (\"\")"), s=w784, f=w792) -> (s? t:f=w790:string)
        n481 = call "Add State to Queue.vi"("State(s) In Front (\"\")"=w790, "State(s) In (\"\")"=w798) -> ("States Out"=w797:string)  [unwired: 13 in]
      }
      frame "质控单元排液中" {
        n482 = case shown="真" w818 {
          tunnel: w819 -> [_ w835]
          tunnel: w821 -> [_ w834]
          frame False {
          }
          frame True {
            n483 = call "启动日志.vi"("日志信息"=w834, "Slave ID"=w835) -> ()  [unwired: 9 in, 1 out]
          }
        }
        n484 = case shown="\"CODCr\"" w819 {
          tunnel: [T12."异常停机" ("运行状态") w837 w839 w841 w843 w845] -> w828
          frame "null", Default {
          }
          frame "氨氮" {
            n485 = global read "ZK非断电保存全局变量.vi" "氨氮质控仪器状态"() -> (w838:T17)
            n486 = Unbundle By Name(w838) -> ("运行状态"=w837:T18)
          }
          frame "总磷" {
            n487 = global read "ZK非断电保存全局变量.vi" "总磷质控仪器状态"() -> (w840:T17)
            n488 = Unbundle By Name(w840) -> ("运行状态"=w839:T18)
          }
          frame "总氮" {
            n489 = global read "ZK非断电保存全局变量.vi" "总氮质控仪器状态"() -> (w842:T17)
            n490 = Unbundle By Name(w842) -> ("运行状态"=w841:T18)
          }
          frame "CODMn" {
            n491 = global read "ZK非断电保存全局变量.vi" "CODMn质控仪器状态"() -> (w844:T17)
            n492 = Unbundle By Name(w844) -> ("运行状态"=w843:T18)
          }
          frame "CODCr" {
            n493 = global read "ZK非断电保存全局变量.vi" "CODCr质控仪器状态"() -> (w846:T17)
            n494 = Unbundle By Name(w846) -> ("运行状态"=w845:T18)
          }
        }
        n495 = Greater Or Equal?(x=w817, y=10) -> (x >= y?=w814:bool)
        n496 = Equal?(x=w828, y=T12."异常停机") -> (x = y?=w820:bool)
        n497 = Equal?(x=w828, y=T12."待机") -> (x = y?=w826:bool)
        n498 = And(x=w814, y=w826) -> (x .and. y?=w815:bool)
        n499 = case shown="真" w820 {
          tunnel: w819 -> [_ w833]
          frame False {
          }
          frame True {
            w832 = "质控单元排液流程中断" ("日志信息")
            n500 = call "启动日志.vi"("日志信息"=w832, "Slave ID"=w833) -> ()  [unwired: 9 in, 1 out]
            n501 = call "报警信息记录.vi"("报警信息"=w832, "Slave ID"=w833) -> ()  [unwired: 9 in, 1 out]
          }
        }
        n502 = Select(t="", s=w815, f=w821) -> (s? t:f=w824:string)
        n503 = Select(t="流程结束" ("State(s) In (\"\")"), s=w820, f=w824) -> (s? t:f=w822:string)
        n504 = call "Add State to Queue.vi"("State(s) In Front (\"\")"=w822, "State(s) In (\"\")"=w831) -> ("States Out"=w830:string)  [unwired: 13 in]
      }
      frame "-------------------# 仪器测试流程 #-------------------" {
        n505 = call "Add State to Queue.vi"("State(s) In (\"\")"=w849) -> ("States Out"=w848:string)  [unwired: 14 in]
      }
      frame "启动仪器水样测试" {
        n506 = Get Date/Time In Seconds() -> (seconds since 1Jan1904=→"水样测试启动时间":timestamp)
        n507 = call "启动日志.vi"("日志信息"=w853, "Slave ID"=w854) -> ()  [unwired: 9 in, 1 out]
        n508 = case shown="\"总氮\"" w854 {
          tunnel: enum16{"水样测试", "平行样测试", "加标回收", "停止"}."水样测试" ("控制命令") -> [_ w863 w864 w865 w866 w867]
          frame "null", Default {
          }
          frame "氨氮" {
            n509 = call "氨氮启动器.vi"("控制命令"=w863) -> ()  [unwired: 11 in]
          }
          frame "总磷" {
            n510 = call "总磷启动器.vi"("控制命令"=w864) -> ()  [unwired: 11 in]
          }
          frame "总氮" {
            n511 = call "总氮启动器.vi"("控制命令"=w865) -> ()  [unwired: 11 in]
          }
          frame "CODMn" {
            n512 = call "CODmn启动器.vi"("控制命令"=w866) -> ()  [unwired: 11 in]
          }
          frame "CODCr" {
            n513 = call "CODcr启动器.vi"("控制命令"=w867) -> ()  [unwired: 11 in]
          }
        }
        n514 = Index Array(array=w857, index=5 ("索引")) -> (element=w856:refnum<vi>)
        n515 = property class="DigNum (严格)"(reference=w856) -> (reference out=w860:refnum<vi>, "Value"=w859:u16)  [unwired: 1 in, 1 out]
        n516 = Increment(x=w859) -> (x+1=w858:u16)
        n517 = property class="DigNum (严格)"(reference=w860, "Value"=w858) -> ()  [unwired: 1 in, 2 out]
        n518 = call "Add State to Queue.vi"("State(s) In (\"\")"=w862) -> ("States Out"=w861:string)  [unwired: 14 in]
      }
      frame "等待仪器空闲" {
        n519 = case shown="真" w868 {
          tunnel: w871 -> [_ w889]
          tunnel: w870 -> [_ w888]
          frame False {
          }
          frame True {
            n520 = call "启动日志.vi"("日志信息"=w888, "Slave ID"=w889) -> ()  [unwired: 9 in, 1 out]
          }
        }
        n521 = case shown="\"总磷\"" w871 {
          tunnel: w870 -> [_ w876]
          tunnel: [_ w875] -> w869
          frame "null", Default {
          }
          frame "总磷" {
            n522 = global read "系统交互.vi" "总磷总氮类型"() -> (w877:enum16{"单模块", "总磷总氮二合一模块", "氨氮总磷二合一模块"})
            n523 = case shown="\"氨氮总磷二合一模块\"" w877 {
              tunnel: w876 -> [_ w880 w885]
              tunnel: [_ w879 w884] -> w875
              frame "单模块", Default {
              }
              frame "总磷总氮二合一模块" {
                n524 = global read "ZK非断电保存全局变量.vi" "流程运行状态标记位"() -> (w882:T6)
                n525 = Unbundle By Name(w882) -> ("总氮"=w881:bool)
                n526 = Select(t=w880, s=w881, f="") -> (s? t:f=w879:string)
              }
              frame "氨氮总磷二合一模块" {
                n527 = global read "ZK非断电保存全局变量.vi" "流程运行状态标记位"() -> (w887:T6)
                n528 = Unbundle By Name(w887) -> ("氨氮"=w886:bool)
                n529 = Select(t=w885, s=w886, f="") -> (s? t:f=w884:string)
              }
            }
          }
        }
        n530 = call "Add State to Queue.vi"("State(s) In Front (\"\")"=w869, "State(s) In (\"\")"=w874) -> ("States Out"=w873:string)  [unwired: 13 in]
      }
      frame "启动仪器加标回收测试" {
        n531 = Get Date/Time In Seconds() -> (seconds since 1Jan1904=→"加标回收启动时间":timestamp)
        n532 = call "启动日志.vi"("日志信息"=w893, "Slave ID"=w894) -> ()  [unwired: 9 in, 1 out]
        n533 = case shown="\"CODMn\"" w894 {
          tunnel: enum16{"水样测试", "平行样测试", "加标回收", "停止"}."加标回收" ("控制命令") -> [_ w903 w904 w905 w906 w907]
          frame "null", Default {
          }
          frame "氨氮" {
            n534 = call "氨氮启动器.vi"("控制命令"=w903) -> ()  [unwired: 11 in]
          }
          frame "总磷" {
            n535 = call "总磷启动器.vi"("控制命令"=w904) -> ()  [unwired: 11 in]
          }
          frame "总氮" {
            n536 = call "总氮启动器.vi"("控制命令"=w905) -> ()  [unwired: 11 in]
          }
          frame "CODMn" {
            n537 = call "CODmn启动器.vi"("控制命令"=w906) -> ()  [unwired: 11 in]
          }
          frame "CODCr" {
            n538 = call "CODcr启动器.vi"("控制命令"=w907) -> ()  [unwired: 11 in]
          }
        }
        n539 = Index Array(array=w897, index=6 ("索引")) -> (element=w896:refnum<vi>)
        n540 = property class="DigNum (严格)"(reference=w896) -> (reference out=w900:refnum<vi>, "Value"=w899:u16)  [unwired: 1 in, 1 out]
        n541 = Increment(x=w899) -> (x+1=w898:u16)
        n542 = property class="DigNum (严格)"(reference=w900, "Value"=w898) -> ()  [unwired: 1 in, 2 out]
        n543 = call "Add State to Queue.vi"("State(s) In (\"\")"=w902) -> ("States Out"=w901:string)  [unwired: 14 in]
      }
      frame "启动仪器平行样测试" {
        n544 = Get Date/Time In Seconds() -> (seconds since 1Jan1904=→"平行样启动时间":timestamp)
        n545 = call "启动日志.vi"("日志信息"=w911, "Slave ID"=w912) -> ()  [unwired: 9 in, 1 out]
        n546 = case shown="\"总磷\"" w912 {
          tunnel: enum16{"水样测试", "平行样测试", "加标回收", "停止"}."平行样测试" ("控制命令") -> [_ w921 w922 w923 w924 w925]
          frame "null", Default {
          }
          frame "氨氮" {
            n547 = call "氨氮启动器.vi"("控制命令"=w921) -> ()  [unwired: 11 in]
          }
          frame "总磷" {
            n548 = call "总磷启动器.vi"("控制命令"=w922) -> ()  [unwired: 11 in]
          }
          frame "总氮" {
            n549 = call "总氮启动器.vi"("控制命令"=w923) -> ()  [unwired: 11 in]
          }
          frame "CODMn" {
            n550 = call "CODmn启动器.vi"("控制命令"=w924) -> ()  [unwired: 11 in]
          }
          frame "CODCr" {
            n551 = call "CODcr启动器.vi"("控制命令"=w925) -> ()  [unwired: 11 in]
          }
        }
        n552 = Index Array(array=w915, index=6 ("索引")) -> (element=w914:refnum<vi>)
        n553 = property class="DigNum (严格)"(reference=w914) -> (reference out=w918:refnum<vi>, "Value"=w917:u16)  [unwired: 1 in, 1 out]
        n554 = Increment(x=w917) -> (x+1=w916:u16)
        n555 = property class="DigNum (严格)"(reference=w918, "Value"=w916) -> ()  [unwired: 1 in, 2 out]
        n556 = call "Add State to Queue.vi"("State(s) In (\"\")"=w920) -> ("States Out"=w919:string)  [unwired: 14 in]
      }
      frame "exit" {
        n557 = call "启动日志.vi"("日志信息"=w930, "Slave ID"=w928) -> ()  [unwired: 9 in, 1 out]
        n558 = flat-sequence {
          tunnel: w928 -> [w933]
          frame #0 {
            n559 = global read "ZK非断电保存全局变量.vi" "流程运行状态标记位"() -> (w934:T6)
            n560 = case shown="\"氨氮\"" w933 {
              tunnel: w934 -> [_ w937 w938 w941 w944 w947]
              frame "null", Default {
              }
              frame "氨氮" {
                n561 = Bundle By Name(cluster=w937, "氨氮"=FALSE) -> (w936:T6)
                n562 = global write "ZK非断电保存全局变量.vi" "流程运行状态标记位"(w936) -> ()
              }
              frame "总磷" {
                n563 = Bundle By Name(cluster=w938, "总磷"=FALSE ("氨氮")) -> (w940:T6)
                n564 = global write "ZK非断电保存全局变量.vi" "流程运行状态标记位"(w940) -> ()
              }
              frame "总氮" {
                n565 = Bundle By Name(cluster=w941, "总氮"=FALSE ("氨氮")) -> (w943:T6)
                n566 = global write "ZK非断电保存全局变量.vi" "流程运行状态标记位"(w943) -> ()
              }
              frame "CODMn" {
                n567 = Bundle By Name(cluster=w944, "CODMn"=FALSE ("氨氮")) -> (w946:T6)
                n568 = global write "ZK非断电保存全局变量.vi" "流程运行状态标记位"(w946) -> ()
              }
              frame "CODCr" {
                n569 = Bundle By Name(cluster=w947, "CODCr"=FALSE ("氨氮")) -> (w949:T6)
                n570 = global write "ZK非断电保存全局变量.vi" "流程运行状态标记位"(w949) -> ()
              }
            }
          }
          frame #1 {
            n571 = global read "ZK非断电保存全局变量.vi" "流程运行状态标记位"() -> (w953:T6)
            n572 = Cluster To Array(cluster=w953) -> (array=w952:bool[])
            n573 = Boolean Array To Number(Boolean array=w952) -> (number=w951:u32)
            n574 = Equal To 0?(x=w951) -> (x = 0?=w950:bool)
            n575 = case shown="真" w950 {
              frame False {
              }
              frame True {
                n576 = call "采配水启动器.vi"("启动/停止命令"=T8."停止") -> ()  [unwired: 10 in, 1 out]
              }
            }
          }
        }
        n577 = case shown="\"CODMn\"" w928 {
          tunnel: enum16{"水样测试", "平行样测试", "加标回收", "停止"}."停止" ("控制命令") -> [_ w955 w956 w957 w958 w959]
          frame "null", Default {
          }
          frame "氨氮" {
            n578 = call "氨氮启动器.vi"("控制命令"=w955) -> ()  [unwired: 11 in]
          }
          frame "总磷" {
            n579 = call "总磷启动器.vi"("控制命令"=w956) -> ()  [unwired: 11 in]
          }
          frame "总氮" {
            n580 = call "总氮启动器.vi"("控制命令"=w957) -> ()  [unwired: 11 in]
          }
          frame "CODMn" {
            n581 = call "CODmn启动器.vi"("控制命令"=w958) -> ()  [unwired: 11 in]
          }
          frame "CODCr" {
            n582 = call "CODcr启动器.vi"("控制命令"=w959) -> ()  [unwired: 11 in]
          }
        }
        n583 = call "Add State to Queue.vi"("State(s) In Front (\"\")"="流程结束" ("State(s) In Front (\"\")"), "State(s) In (\"\")"=w932) -> ("States Out"=w931:string)  [unwired: 13 in]
      }
      frame "判断仪器水样是否启动成功" {
        n584 = case shown="真" w965 {
          tunnel: w969 -> [_ w985]
          tunnel: w966 -> [_ w984]
          frame False {
          }
          frame True {
            n585 = call "启动日志.vi"("日志信息"=w984, "Slave ID"=w985) -> ()  [unwired: 9 in, 1 out]
          }
        }
        n586 = case shown="\"CODCr\"" w969 {
          tunnel: [T13."空闲" ("工作状态") w990 w992 w994 w996 w998] -> w981
          frame "null", Default {
          }
          frame "氨氮" {
            w989 = u16 3 items=["总磷"=1, "总氮"=2, "氨氮"=3, "CODMn"=21] ("站号")
            n587 = call "获取仪器仪表状态.vi"("站号"=w989) -> ("工作状态"=w990:T13)  [unwired: 10 in]
          }
          frame "总磷" {
            w991 = u16 1 items=["总磷"=1, "总氮"=2, "氨氮"=3, "CODMn"=21] ("站号")
            n588 = call "获取仪器仪表状态.vi"("站号"=w991) -> ("工作状态"=w992:T13)  [unwired: 10 in]
          }
          frame "总氮" {
            w993 = u16 2 items=["总磷"=1, "总氮"=2, "氨氮"=3, "CODMn"=21] ("站号")
            n589 = call "获取仪器仪表状态.vi"("站号"=w993) -> ("工作状态"=w994:T13)  [unwired: 10 in]
          }
          frame "CODMn" {
            w995 = u16 21 items=["总磷"=1, "总氮"=2, "氨氮"=3, "CODMn"=21] ("站号")
            n590 = call "获取仪器仪表状态.vi"("站号"=w995) -> ("工作状态"=w996:T13)  [unwired: 10 in]
          }
          frame "CODCr" {
            w997 = u16 22 items=["总磷"=1, "总氮"=2, "氨氮"=3, "CODMn"=21, "CODcr"=22] ("站号")
            n591 = call "获取仪器仪表状态.vi"("站号"=w997) -> ("工作状态"=w998:T13)  [unwired: 10 in]
          }
        }
        n592 = Index Array(array=w974, index=5 ("索引")) -> (element=w973:refnum<vi>)
        n593 = Greater Or Equal?(x=w968, y=60) -> (x >= y?=w961:bool)
        n594 = property class="DigNum (严格)"(reference=w973) -> ("Value"=w972:u16)  [unwired: 1 in, 2 out]
        n595 = Greater Or Equal?(x=w972, y=u16 5) -> (x >= y?=w970:bool)
        n596 = Equal?(x=w981, y=T13."空闲") -> (x = y?=w962:bool)
        n597 = And(x=w961, y=w962) -> (x .and. y?=w960:bool)
        n598 = case shown="真" w960 {
          tunnel: w969 -> [_ w987]
          frame False {
          }
          frame True {
            w986 = "水样测试启动失败" ("日志信息")
            n599 = call "启动日志.vi"("日志信息"=w986, "Slave ID"=w987) -> ()  [unwired: 9 in, 1 out]
            n600 = call "报警信息记录.vi"("报警信息"=w986, "Slave ID"=w987) -> ()  [unwired: 9 in, 1 out]
          }
        }
        n601 = Select(t="启动仪器水样测试\n判断仪器水样是否启动成功" ("State(s) In (\"\")"), s=w962, f="") -> (s? t:f=w964:string)
        n602 = Select(t=w964, s=w961, f=w966) -> (s? t:f=w963:string)
        n603 = Select(t="流程结束" ("State(s) In (\"\")"), s=w970, f=w963) -> (s? t:f=w975:string)
        n604 = call "Add State to Queue.vi"("State(s) In Front (\"\")"=w975, "State(s) In (\"\")"=w983) -> ("States Out"=w982:string)  [unwired: 13 in]
      }
      frame "判断仪器加标是否启动成功" {
        n605 = case shown="真" w1005 {
          tunnel: w1004 -> [_ w1024]
          tunnel: w1008 -> [_ w1023]
          frame False {
          }
          frame True {
            n606 = call "启动日志.vi"("日志信息"=w1024, "Slave ID"=w1023) -> ()  [unwired: 9 in, 1 out]
          }
        }
        n607 = case shown="\"CODCr\"" w1008 {
          tunnel: [T13."空闲" ("工作状态") w1029 w1031 w1033 w1035 w1037] -> w1010
          frame "null", Default {
          }
          frame "氨氮" {
            w1028 = u16 3 items=["总磷"=1, "总氮"=2, "氨氮"=3, "CODMn"=21] ("站号")
            n608 = call "获取仪器仪表状态.vi"("站号"=w1028) -> ("工作状态"=w1029:T13)  [unwired: 10 in]
          }
          frame "总磷" {
            w1030 = u16 1 items=["总磷"=1, "总氮"=2, "氨氮"=3, "CODMn"=21] ("站号")
            n609 = call "获取仪器仪表状态.vi"("站号"=w1030) -> ("工作状态"=w1031:T13)  [unwired: 10 in]
          }
          frame "总氮" {
            w1032 = u16 2 items=["总磷"=1, "总氮"=2, "氨氮"=3, "CODMn"=21] ("站号")
            n610 = call "获取仪器仪表状态.vi"("站号"=w1032) -> ("工作状态"=w1033:T13)  [unwired: 10 in]
          }
          frame "CODMn" {
            w1034 = u16 21 items=["总磷"=1, "总氮"=2, "氨氮"=3, "CODMn"=21] ("站号")
            n611 = call "获取仪器仪表状态.vi"("站号"=w1034) -> ("工作状态"=w1035:T13)  [unwired: 10 in]
          }
          frame "CODCr" {
            w1036 = u16 22 items=["总磷"=1, "总氮"=2, "氨氮"=3, "CODMn"=21, "CODcr"=22] ("站号")
            n612 = call "获取仪器仪表状态.vi"("站号"=w1036) -> ("工作状态"=w1037:T13)  [unwired: 10 in]
          }
        }
        n613 = Index Array(array=w1014, index=6 ("索引")) -> (element=w1013:refnum<vi>)
        n614 = Greater Or Equal?(x=w1007, y=60) -> (x >= y?=w1000:bool)
        n615 = property class="DigNum (严格)"(reference=w1013) -> ("Value"=w1012:u16)  [unwired: 1 in, 2 out]
        n616 = Greater Or Equal?(x=w1012, y=u16 5) -> (x >= y?=w1009:bool)
        n617 = Equal?(x=w1010, y=T13."空闲") -> (x = y?=w1001:bool)
        n618 = And(x=w1000, y=w1001) -> (x .and. y?=w999:bool)
        n619 = case shown="真" w999 {
          tunnel: w1008 -> [_ w1026]
          frame False {
          }
          frame True {
            w1025 = "加标回收启动失败" ("日志信息")
            n620 = call "启动日志.vi"("日志信息"=w1025, "Slave ID"=w1026) -> ()  [unwired: 9 in, 1 out]
            n621 = call "报警信息记录.vi"("报警信息"=w1025, "Slave ID"=w1026) -> ()  [unwired: 9 in, 1 out]
          }
        }
        n622 = Select(t="启动仪器加标回收测试\n判断仪器加标是否启动成功" ("State(s) In (\"\")"), s=w1001, f="") -> (s? t:f=w1003:string)
        n623 = Select(t=w1003, s=w1000, f=w1004) -> (s? t:f=w1002:string)
        n624 = Select(t="流程结束" ("State(s) In (\"\")"), s=w1009, f=w1002) -> (s? t:f=w1015:string)
        n625 = call "Add State to Queue.vi"("State(s) In Front (\"\")"=w1015, "State(s) In (\"\")"=w1022) -> ("States Out"=w1021:string)  [unwired: 13 in]
      }
      frame "判断仪器平行样是否启动成功" {
        n626 = case shown="真" w1043 {
          tunnel: w1047 -> [_ w1063]
          tunnel: w1044 -> [_ w1062]
          frame False {
          }
          frame True {
            n627 = call "启动日志.vi"("日志信息"=w1062, "Slave ID"=w1063) -> ()  [unwired: 9 in, 1 out]
          }
        }
        n628 = case shown="\"CODCr\"" w1047 {
          tunnel: [T13."空闲" ("工作状态") w1068 w1070 w1072 w1074 w1076] -> w1049
          frame "null", Default {
          }
          frame "氨氮" {
            w1067 = u16 3 items=["总磷"=1, "总氮"=2, "氨氮"=3, "CODMn"=21] ("站号")
            n629 = call "获取仪器仪表状态.vi"("站号"=w1067) -> ("工作状态"=w1068:T13)  [unwired: 10 in]
          }
          frame "总磷" {
            w1069 = u16 1 items=["总磷"=1, "总氮"=2, "氨氮"=3, "CODMn"=21] ("站号")
            n630 = call "获取仪器仪表状态.vi"("站号"=w1069) -> ("工作状态"=w1070:T13)  [unwired: 10 in]
          }
          frame "总氮" {
            w1071 = u16 2 items=["总磷"=1, "总氮"=2, "氨氮"=3, "CODMn"=21] ("站号")
            n631 = call "获取仪器仪表状态.vi"("站号"=w1071) -> ("工作状态"=w1072:T13)  [unwired: 10 in]
          }
          frame "CODMn" {
            w1073 = u16 21 items=["总磷"=1, "总氮"=2, "氨氮"=3, "CODMn"=21] ("站号")
            n632 = call "获取仪器仪表状态.vi"("站号"=w1073) -> ("工作状态"=w1074:T13)  [unwired: 10 in]
          }
          frame "CODCr" {
            w1075 = u16 22 items=["总磷"=1, "总氮"=2, "氨氮"=3, "CODMn"=21, "CODcr"=22] ("站号")
            n633 = call "获取仪器仪表状态.vi"("站号"=w1075) -> ("工作状态"=w1076:T13)  [unwired: 10 in]
          }
        }
        n634 = Index Array(array=w1053, index=6 ("索引")) -> (element=w1052:refnum<vi>)
        n635 = Greater Or Equal?(x=w1046, y=60) -> (x >= y?=w1039:bool)
        n636 = property class="DigNum (严格)"(reference=w1052) -> ("Value"=w1051:u16)  [unwired: 1 in, 2 out]
        n637 = Greater Or Equal?(x=w1051, y=u16 5) -> (x >= y?=w1048:bool)
        n638 = Equal?(x=w1049, y=T13."空闲") -> (x = y?=w1040:bool)
        n639 = And(x=w1039, y=w1040) -> (x .and. y?=w1038:bool)
        n640 = case shown="真" w1038 {
          tunnel: w1047 -> [_ w1065]
          frame False {
          }
          frame True {
            w1064 = "平行样启动失败" ("日志信息")
            n641 = call "启动日志.vi"("日志信息"=w1064, "Slave ID"=w1065) -> ()  [unwired: 9 in, 1 out]
            n642 = call "报警信息记录.vi"("报警信息"=w1064, "Slave ID"=w1065) -> ()  [unwired: 9 in, 1 out]
          }
        }
        n643 = Select(t="启动仪器平行样测试\n判断仪器平行样是否启动成功" ("State(s) In (\"\")"), s=w1040, f="") -> (s? t:f=w1042:string)
        n644 = Select(t=w1042, s=w1039, f=w1044) -> (s? t:f=w1041:string)
        n645 = Select(t="流程结束" ("State(s) In (\"\")"), s=w1048, f=w1041) -> (s? t:f=w1054:string)
        n646 = call "Add State to Queue.vi"("State(s) In Front (\"\")"=w1054, "State(s) In (\"\")"=w1061) -> ("States Out"=w1060:string)  [unwired: 13 in]
      }
      frame "仪器加标回收测试中", "仪器平行样测试中", "仪器水样测试中" {
        n647 = case shown="真" w1081 {
          tunnel: w1083 -> [_ w1103]
          tunnel: w1084 -> [_ w1102]
          frame False {
          }
          frame True {
            n648 = call "启动日志.vi"("日志信息"=w1102, "Slave ID"=w1103) -> ()  [unwired: 9 in, 1 out]
          }
        }
        n649 = case shown="\"CODCr\"" w1083 {
          tunnel: [T13."空闲" ("工作状态") w1093 w1095 w1097 w1099 w1101] -> w1082
          frame "null", Default {
          }
          frame "氨氮" {
            w1092 = u16 3 items=["总磷"=1, "总氮"=2, "氨氮"=3, "CODMn"=21] ("站号")
            n650 = call "获取仪器仪表状态.vi"("站号"=w1092) -> ("工作状态"=w1093:T13)  [unwired: 10 in]
          }
          frame "总磷" {
            w1094 = u16 1 items=["总磷"=1, "总氮"=2, "氨氮"=3, "CODMn"=21] ("站号")
            n651 = call "获取仪器仪表状态.vi"("站号"=w1094) -> ("工作状态"=w1095:T13)  [unwired: 10 in]
          }
          frame "总氮" {
            w1096 = u16 2 items=["总磷"=1, "总氮"=2, "氨氮"=3, "CODMn"=21] ("站号")
            n652 = call "获取仪器仪表状态.vi"("站号"=w1096) -> ("工作状态"=w1097:T13)  [unwired: 10 in]
          }
          frame "CODMn" {
            w1098 = u16 21 items=["总磷"=1, "总氮"=2, "氨氮"=3, "CODMn"=21] ("站号")
            n653 = call "获取仪器仪表状态.vi"("站号"=w1098) -> ("工作状态"=w1099:T13)  [unwired: 10 in]
          }
          frame "CODCr" {
            w1100 = u16 22 items=["总磷"=1, "总氮"=2, "氨氮"=3, "CODMn"=21, "CODcr"=22] ("站号")
            n654 = call "获取仪器仪表状态.vi"("站号"=w1100) -> ("工作状态"=w1101:T13)  [unwired: 10 in]
          }
        }
        n655 = Greater Or Equal?(x=w1080, y=30) -> (x >= y?=w1077:bool)
        n656 = Equal?(x=w1082, y=T13."空闲") -> (x = y?=w1087:bool)
        n657 = And(x=w1077, y=w1087) -> (x .and. y?=w1078:bool)
        n658 = Select(t="", s=w1078, f=w1084) -> (s? t:f=w1085:string)
        n659 = call "Add State to Queue.vi"("State(s) In Front (\"\")"=w1085, "State(s) In (\"\")"=w1090) -> ("States Out"=w1089:string)  [unwired: 13 in]
      }
    }
  }
